vi "RT_VS50_Dynamics_DLR_v10_v11_PXI.vi"() -> ()   [LabVIEW 2017]
uses:
  <vilib>/Platform/TimedLoop/XDataNode/timing_clust.ctl
  <vilib>/Platform/TimedLoop/XDataNode/nitl_modes.ctl
  <vilib>/Platform/TimedLoop/XDataNode/wakeup.ctl
  <vilib>/Analysis/coordinate.llb/Euler Rotation Order.ctl
  <vilib>/Analysis/_algsub.llb/Vector Norm Type.ctl
  <vilib>/Analysis/baseanly.llb/Real A x B.vi
  <vilib>/Analysis/_algsub.llb/Real Vector Norm.vi
  <vilib>/Utility/file.llb/Read Delimited Spreadsheet (DBL).vi
  <vilib>/Instr/_visa.llb/VISA Configure Serial Port (Instr).vi
  <vilib>/Analysis/Matrix/Numeric/Conversions/Array To Matrix - RA.vi
  <vilib>/Analysis/Matrix/Numeric/Conversions/Array To Matrix - RA2.vi
  <vilib>/Analysis/Matrix/Numeric/Conversions/Matrix To Array - RM.vi
  <vilib>/Platform/TimedLoop/XDataNode/XDataNode.xnode
  <vilib>/Analysis/NI_AALPro.lvlib
  <vilib>/Platform/TimedLoop/XDataNode/XDNodeRunTimeDep.lvlib
  <vilib>/Utility/file.llb/Read From Spreadsheet File (DBL).vi
  <vilib>/Analysis/Matrix/NI_Matrix.lvlib
  <vilib>/Analysis/NI_AALBase.lvlib
panel:
  out "Sim_Time [s]":dbl
  in  "Simulation Parameters":T1={"Wind VelocityAzimuth [deg] "=0.0, "Wind Velocity Module [m/s]"=0.0, "Fe gain"=1.0, "Cnalpha gain"=1.0, "clp gain"=1.0, "cld gain"=1.0, "cmq gain"=1.0, "cnr gain"=1.0, "dl [º]"=0.0, "Nozzle misalignment yaw/pitch [º]"=[0.0, 0.0], "Nozzle eccentricity x/y [m]"=[], "Wind_Profile"=0} {"Wind_Profile" min=0 max=3 step=1; "Wind Velocity Module [m/s]" format="%#_13g"; "Wind VelocityAzimuth [deg]" format="%#_13g"}
  in  "Initialization Parameters":T2={"W_b ini [rad/s]"=[0.0, 0.0, 0.0], "W ini [rad/s]"=[0.0, 0.0, 0.0], "altitude_ini(m)"=50.0, "lon_ini [º]"=-44.36778, "latd_ini [º]"=-2.31599, "V_ini [m/s]"=[0.0, 0.0, 0.0], "Initial Euler Angles [deg]"=[0.0, 0.0, 0.0], "CFN-61G Enable"=FALSE, "Table enable"=FALSE, "DMARS Enable"=FALSE, "TVA Enable"=FALSE, "Sim_Time [s]"=82.0, "Control Selection"=enum."Sim Control"}
  in  "Rotation":T3
  out "Initial Euler Angles [deg] 2":cluster{"phi":dbl, "theta":dbl, "psi":dbl}
  out "TVA_cmd [deg] 2":dbl[](array[numeric])
  out "Control Variables (extra variables)":dbl[](array[numeric])
  in  "Send":bool
  out "Table Ready":bool
  out "CIVITA as DMARS [º]":cluster{"phi":dbl, "theta":dbl, "psi":dbl}
  in  "Cluster":T4={"Offset Roll"=0.0, "Offset Pitch"=0.0, "Offset Heading"=0.0, "Azimuth"=0.0, "Latitude "=-23.213156, "Longitude"=-45.860622, "Height"=622.367, "LP_Vel_Z-North"=0.0, "LP_Vel_Y-East"=0.0, "LP_Vel_X-Up"=0.0}
  out "Table cmd [º] inner middle outer":dbl[](array[numeric])
  out "DMARS SIM pred[º]":cluster{"phi":dbl, "theta":dbl, "psi":dbl}
  out "Control Variables\n (extra variables)":dbl[](array[numeric])
  out "ACT 315 Angle \"Yaw\"":dbl(slide) scale=-3.0..3.0
  out "ACT 225 Angle \"Pitch\"":dbl(slide) scale=-3.0..3.0
  out "TVA string 2":string
  out "TVA bytes read 2":u32
  out "CRC Check over Byte #10 to byte #84":bool
  out "CRC Check over Byte #2 to Byte #7 TVA2BComp":bool
  out "Iteration Duration":i64
  out "Roll Rate/angle":dbl[](array[numeric])
  out "CRC Check over Byte #2 to Byte #7":bool
  out "CRC Check over Byte #10 to byte #29":bool
  out "GC_Counter 2":u32
  out "concatenated string 2":string
  out "PXI log path 2":path
  out "string to write DMARS":string="*IDN?"
  out "TVA string":string
  out "TVA bytes read":u32
  out "TVA sync bytes":string
  out "read buffer":string
  out "concatenated string":string
  out "appended path":path
  in  "UTC format":bool
  out "spreadsheet string":string
  out "Time (s)":dbl
  out "POS":cluster{dbl, dbl, dbl} {"?" format="%_6g"; "?" format="%#1_6g"}
  out "RATE":cluster{dbl, dbl, dbl} {"?" format="%1_6g"}
  out "ACCEL":cluster{dbl, dbl, dbl} {"?" format="%1_6g"}
  out "Period":i64
  in  "predicted step":dbl=0.04 format="%#_13g"
  out "string enviada para acutrol":string
  in  "Remote Host":string="192.168.53.1"
  out "XYZ - rate_CIVITA":sgl[](array[numeric])
  out "Opp_Mode_CIVITA":string
  in  "NavOn":bool
  in  "Init":bool
  out "read Config port":string
  out "Long_Lat_Alt_CIVITA":sgl[](array[numeric])
  out "Euler Angles_CIVITA":sgl[](array[numeric])
  out "all rows":dbl[][](array[numeric]) format="%0.3f"
  in  "Run_SIMULATION":bool
  out "Data 4":dbl[][](array[numeric])
  out "Data 3":dbl[][](array[numeric])
  out "Data 2":dbl[][](array[numeric])
  out "Iteration Duration [us]":i64(graph)
  out "Current time [s]":dbl
  out "TVA_cmd [deg]":dbl[](array[numeric])
  out "bad iteration":bool
  in  "stop RT":bool
  out "SIM_Running":bool
  # "atitudes após leveling"
  # "INS Civitanavi Control"
  # "0.279817"
  # "0.24729"
  # "0.119821"
  # "-0.038247"
  # "0xAA/ 0x55"
  # "-0.038932"
  # "-0.0385253"
  # "-0.0178696"
  # "-0.0193609"
  # "-0.0176574"
  # "830 steps"
  # "Posicão inicial"
  # "Posicao after 10min"
  # "-48.1427"
  # "-45.8606"
  # "-23.2324"
  # "-23.2132"
  # "-4.67869"
  # "0.622374"
  # "º"
  # "º"
  # "Km"
  # "Simulation"
  # "Motion simulation table Control and Log files"
  # "Reiniciar a vi sempre antes de uma nova simulação!!"
  # "0.766"
  # "1.532"
  # "Enable buttons"
  # "TVA COMMUNICATIONS"
  # "0.643"
  # "1.286"
  # "Housekeeping data"
  # "Command Data"
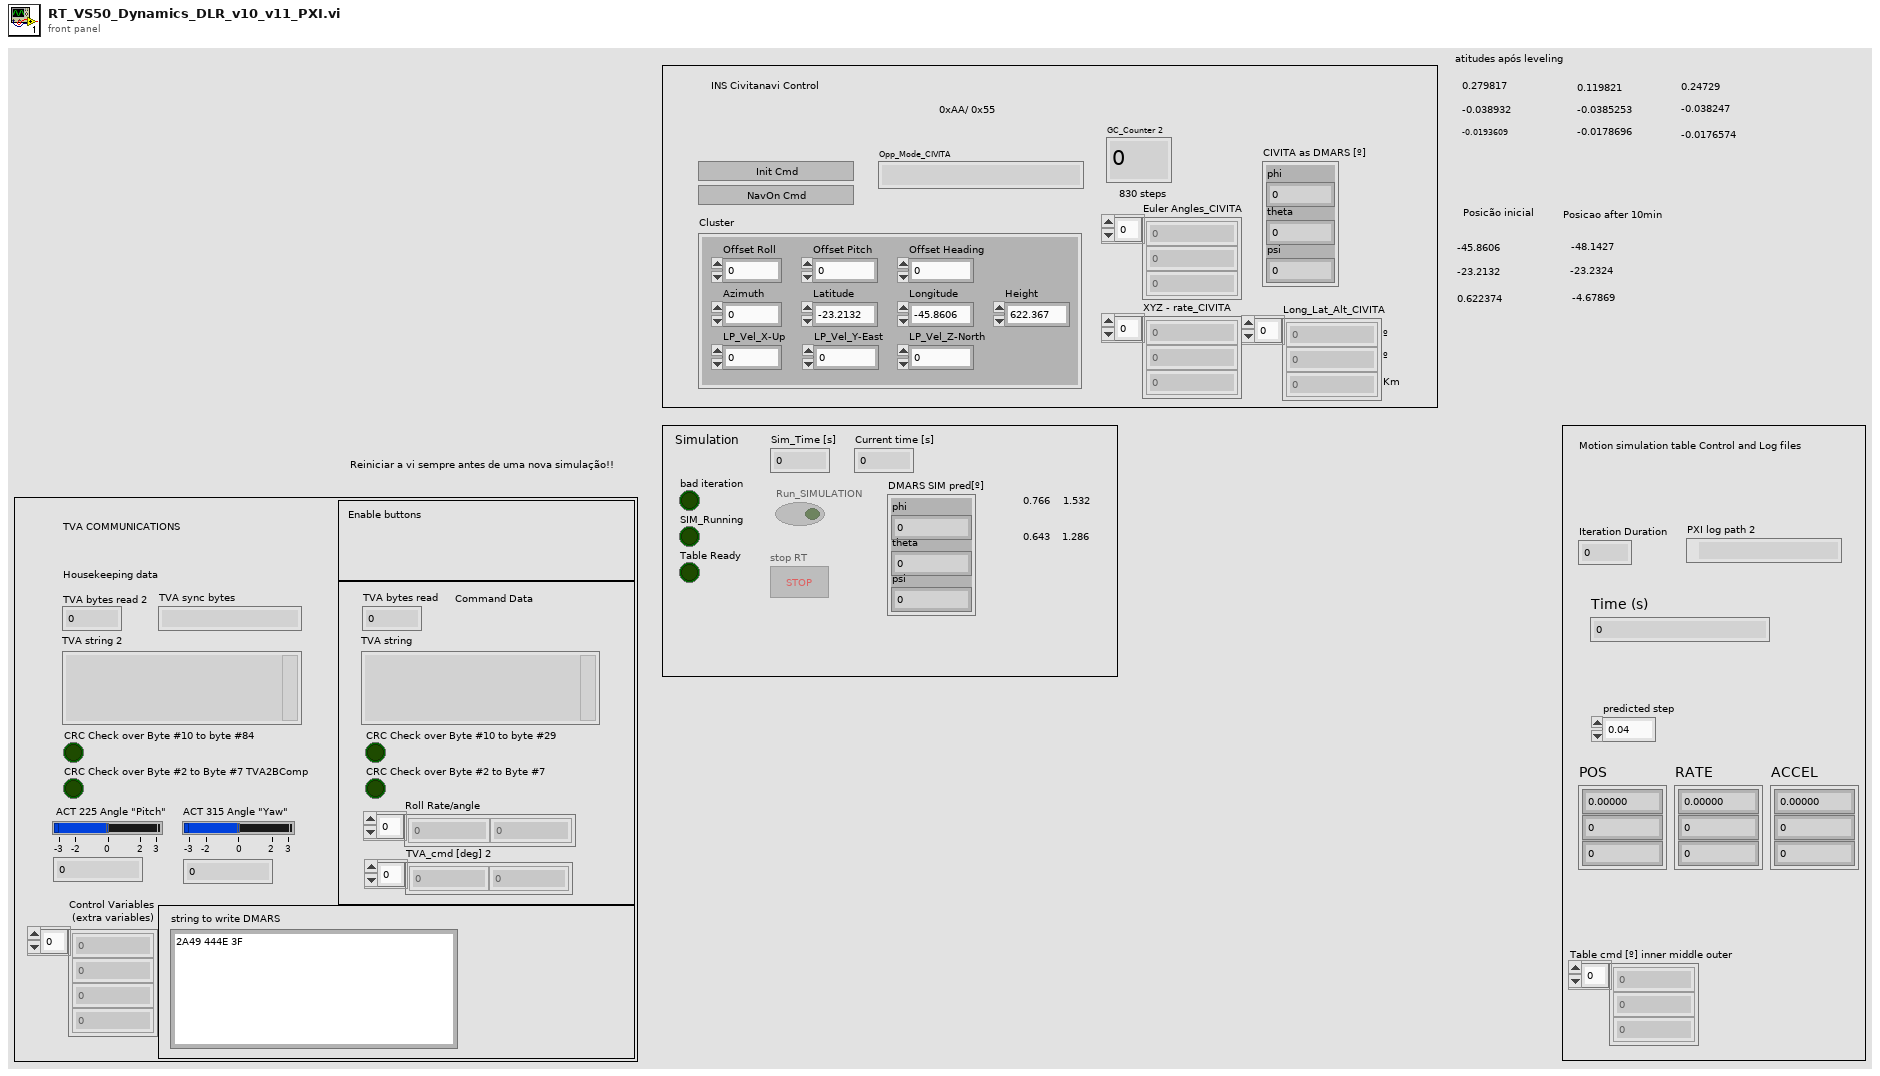
[diagram p1: front panel]
types:
  T1 = cluster{"Wind VelocityAzimuth [deg] ":dbl, "Wind Velocity Module [m/s]":dbl, "Fe gain":dbl, "Cnalpha gain":dbl, "clp gain":dbl, "cld gain":dbl, "cmq gain":dbl, "cnr gain":dbl, "dl [º]":dbl, "Nozzle misalignment yaw/pitch [º]":dbl[], "Nozzle eccentricity x/y [m]":dbl[], "Wind_Profile":i32}
  T2 = cluster{"W_b ini [rad/s]":dbl[], "W ini [rad/s]":dbl[], "altitude_ini(m)":dbl, "lon_ini [º]":dbl, "latd_ini [º]":dbl, "V_ini [m/s]":dbl[], "Initial Euler Angles [deg]":dbl[], "CFN-61G Enable":bool, "Table enable":bool, "DMARS Enable":bool, "TVA Enable":bool, "Sim_Time [s]":dbl, "Control Selection":enum16{"Constant", "TVA E-BOX", "Sim Control"}}
  T3 = cluster{"W(i) [rad/s]":dbl[], "W_b(i) [rad/s]":dbl[], "q(i)":dbl[], "Euler Angles {rad]":dbl[]}
  T4 = cluster{"Offset Roll":sgl, "Offset Pitch":sgl, "Offset Heading":sgl, "Azimuth":sgl, "Latitude ":sgl, "Longitude":sgl, "Height":sgl, "LP_Vel_Z-North":sgl, "LP_Vel_Y-East":sgl, "LP_Vel_X-Up":sgl}
  T5 = typedef "XDNodeRunTimeDep.lvlib/timing_clust.ctl" = cluster{"Expected End [f-1]":u64, "Actual End [f-1]":u64, "Finished Late? [f-1]":bool, "Expected End [i-1]":u64, "Actual End [i-1]":u64, "Finished Late? [i-1]":bool, "Expected Start [i]":u64, "Actual Start [i]":u64, "Expected Start [f]":u64, "Actual Start [f]":u64, "Source Name":string, "Structure Name":string, "Period":i64, "Deadline":i64, "Offset":i64, "Start":i64, "Priority":i32, "Timeout":i32, "Mode":T6, "Wakeup Reason":T7, "Error":errorcluster, "Source Type":string, "Secondary Source Type":string, "Global End Time":u64, "Global Start Time":u64, "Frame Duration":u64, "Iteration Duration":u64, "Assigned CPU":i32, "I/O Scan Engine Mode":u32}
  T6 = typedef "XDNodeRunTimeDep.lvlib/nitl_modes.ctl" = enum32{"No Change", "Process missed periods, maintain original phase", "Discard missed periods, maintain original phase", "Process missed periods, ignore original phase", "Discard missed periods, ignore original phase"}
  T7 = typedef "XDNodeRunTimeDep.lvlib/wakeup.ctl" = enum32{"Normal", "Aborted", "Asynchronous wakeup", "Timing source error", "Timed loop error", "Timeout"}
  T8 = cluster{"act_b [rad]":dbl[], "Oil Consumption [L]":dbl, "Act_b_TVA (315,225) [deg]":dbl[]}
  T9 = cluster{"W(i+1) [rad/s]":dbl[], "W_b(i+1) [rad/s]":dbl[], "q(i+1)":dbl[], "Euler angles (i+1) XYZ [rad]":dbl[]}
  T10 = cluster{"position ECEF (i)":dbl[], "Lat_C [rad]":dbl, "latd(i+1) [rad]":dbl, "lon(i+1) [rad]":dbl, "height (i+1) [m]":dbl, "V(i+1) [m/s] NWU":dbl[]}
  T11 = cluster{"latd(i) [rad]":dbl, "lon(i) [rad]":dbl, "height(i)(m)":dbl, "V(i) [m/s] NWU":dbl[]}
  T12 = typedef "NI_AALPro.lvlib/Euler Rotation Order.ctl" = u16
  T13 = cluster{"dt [s]":dbl, "sim_running":bool, "t[s]":dbl, "i":i32}
  T14 = cluster{"Nzl_S [m^2]":dbl, "le [m]":dbl, "dl [rad]":dbl, "Dref[m]":dbl, "Sref [m^2]":dbl, "Nozzle misalignment yaw/pitch [º]":dbl[], "Nozzle eccentricity x/y [m]":dbl[]}
  T15 = typedef "NI_Matrix.lvlib/RealMatrix.ctl" = dbl[][]
  T16 = cluster{"AoA_pitch [rad]":dbl, "AoA_yaw [rad]":dbl, "Stream_direction [rad]":dbl[], "Speed_direction [rad]":dbl[]}
  T17 = cluster{"M_alpha [rad/s²]":dbl, "M_beta [rad/s²]":dbl}
  T18 = typedef "NI_AALPro.lvlib/Vector Norm Type.ctl" = u16
  T19 = enum16{"open", "replace", "create", "open or create", "replace or create", "replace or create with confirmation"}
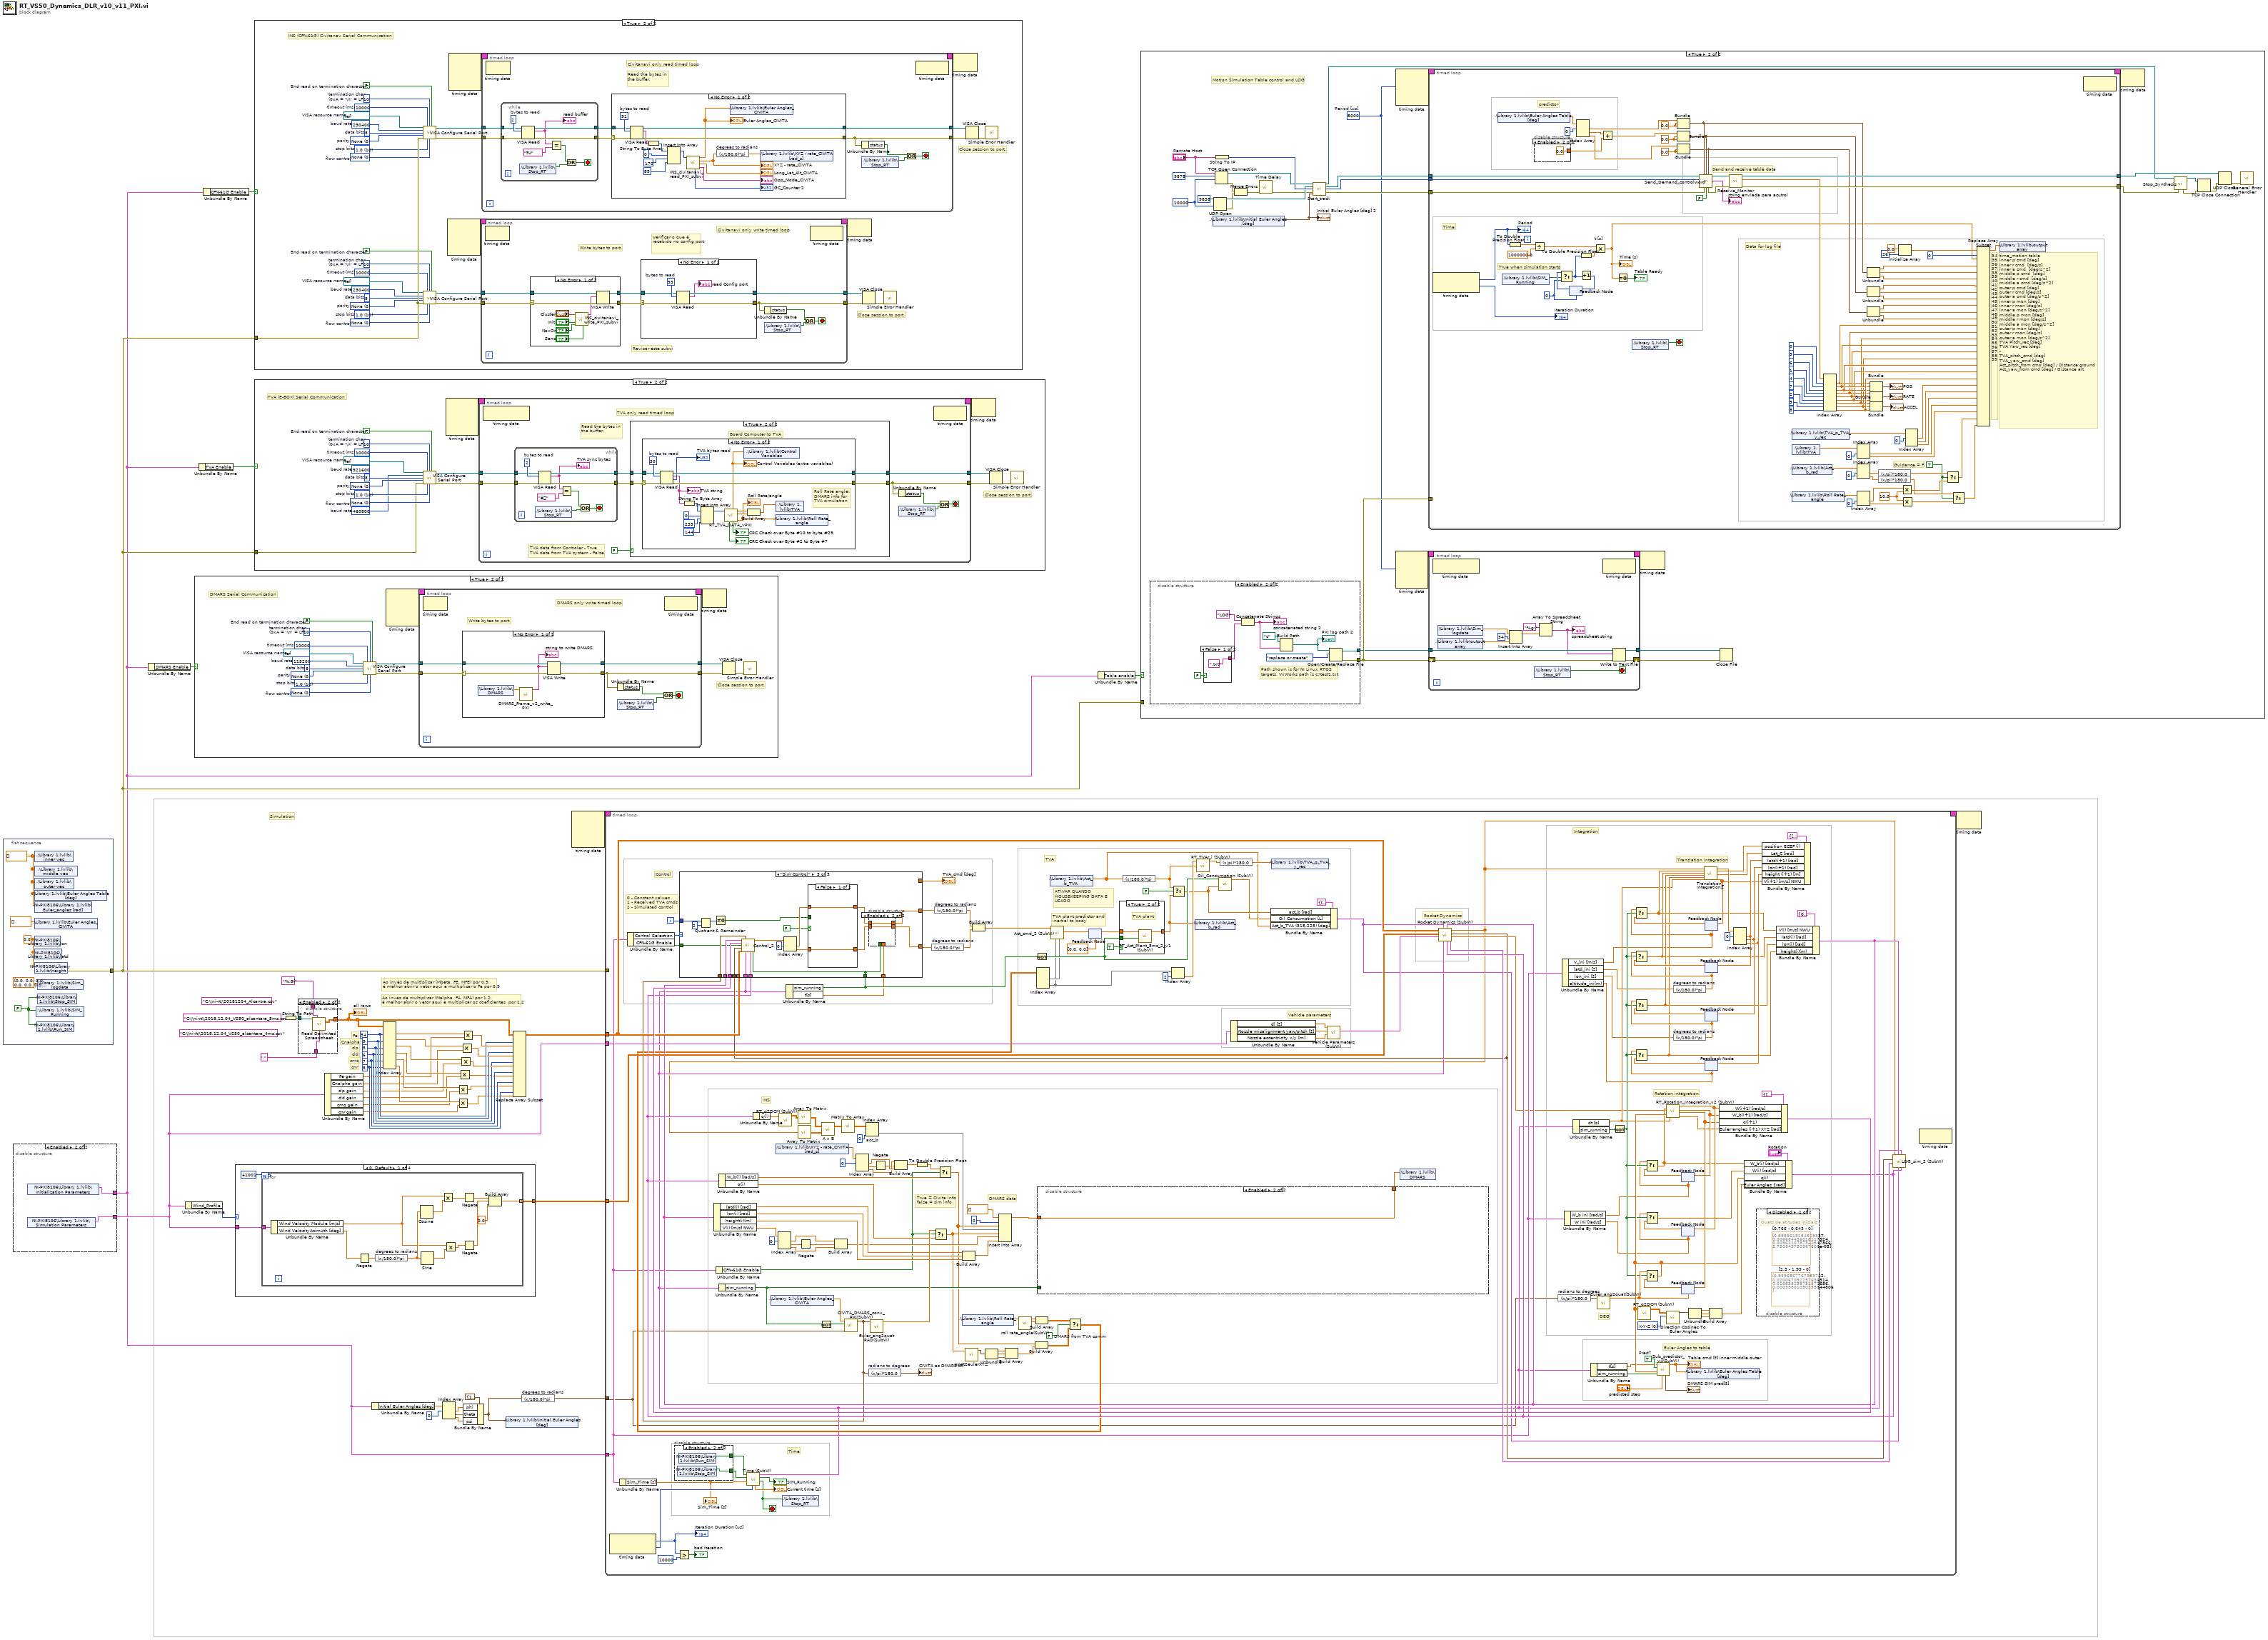
[diagram p0: block diagram]
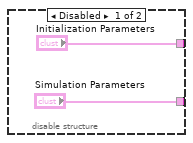
[diagram p2: hidden frame]
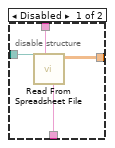
[diagram p3: hidden frame]
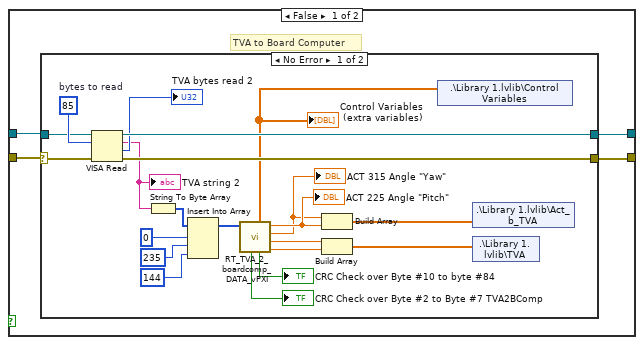
[diagram p11: hidden frame]
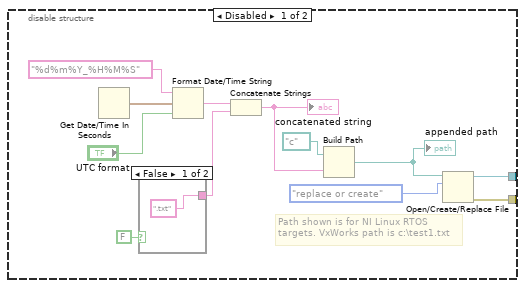
[diagram p15: hidden frame]
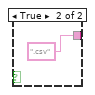
[diagram p16: hidden frame]
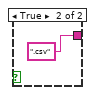
[diagram p17: hidden frame]
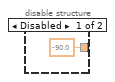
[diagram p18: hidden frame]
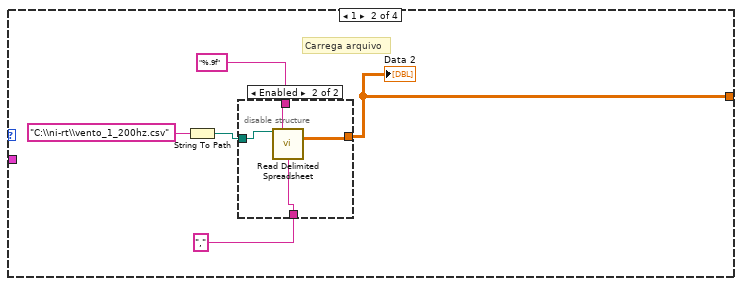
[diagram p19: hidden frame]
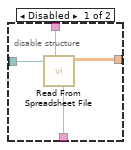
[diagram p20: hidden frame]
diagram:
  w27 = 8 ("index (col)")
  w28 = 7 ("index (col)")
  w29 = 6 ("index (col)")
  w33 = 5 ("index (col)")
  w36 = 9 ("index (col)")
  w41 = 54 ("disabled index (col)")
  (unwired) "C:\\ni-rt\\2018.12.04_VS50_alcantara_4ms.csv"
  (unwired) "C:\\ni-rt\\20181204_Alcantra.csv"
  # "cnr"
  # "cmq"
  # "cld"
  # "clp"
  # "Cnalpha"
  # "Fe"
  # "Ao invés de multiplicar (Malpha, FA, MFA) por 1.2,\né melhor abrir o vetor aqui e multiplicar os coeficientes  por 1.2"
  # "Ao invés de multiplicar (Mbeta, FE, MFE) por 0.9,\né melhor abrir o vetor aqui e multiplicar o Fe por 0.9"
  # "Simulation"
  n1 = flat-sequence {
    tunnel: [w53] -> w22
    frame #0 {
      w52 = dbl[] [] ("inner vec")
      w50 = FALSE ("SIM_Running")
      w55 = 0.0 ("lon")
      n2 = shared-variable ".\\Library 1.lvlib\\inner vec"(w52) -> ()  [unwired: 1 in, 1 out]
      n3 = shared-variable ".\\Library 1.lvlib\\middle vec"(w52) -> ()  [unwired: 1 in, 1 out]
      n4 = shared-variable ".\\Library 1.lvlib\\outer vec"(w52) -> ()  [unwired: 1 in, 1 out]
      n5 = shared-variable ".\\Library 1.lvlib\\Euler Angles Table [deg]"(w52) -> ()  [unwired: 1 in, 1 out]
      n6 = shared-variable "NI-PXI8106\\Library 1.lvlib\\Euler_angles [rad]"(w52) -> ()  [unwired: 1 in, 1 out]
      n7 = shared-variable ".\\Library 1.lvlib\\Euler Angles_CIVITA"(sgl[] [] ("Euler Angles_CIVITA")) -> ()  [unwired: 1 in, 1 out]
      n8 = shared-variable "NI-PXI8106\\Library 1.lvlib\\lon"(w55) -> ()  [unwired: 1 in, 1 out]
      n9 = shared-variable "NI-PXI8106\\Library 1.lvlib\\latd"(w55) -> ()  [unwired: 1 in, 1 out]
      n10 = shared-variable "NI-PXI8106\\Library 1.lvlib\\height"(w55) -> (error out=w53:errorcluster)  [unwired: 1 in]
      n11 = shared-variable ".\\Library 1.lvlib\\SIM_Running"(w50) -> ()  [unwired: 1 in, 1 out]
      n12 = shared-variable "NI-PXI8106\\Library 1.lvlib\\Run_SIM"(w50) -> ()  [unwired: 1 in, 1 out]
      n13 = shared-variable ".\\Library 1.lvlib\\Sim_logdata"(dbl[] [0.0, 0.0, 0.0, 0.0, 0.0, 0.0, 0.0, 0.0, 0.0, 0.0, 0.0, 0.0, 0.0, 0.0, 0.0, 0.0, 0.0, 0.0, 0.0, 0.0, 0.0, 0.0, 0.0, 0.0, 0.0, 0.0, 0.0, 0.0, 0.0, 0.0, 0.0, 0.0, 0.0] ("Sim_logdata")) -> ()  [unwired: 1 in, 1 out]
      n14 = shared-variable "NI-PXI8106\\Library 1.lvlib\\Stop_SIM"(w50) -> ()  [unwired: 1 in, 1 out]
    }
  }
  n15 = disable-structure shown="Enabled" {
    disable-tunnel: ["Initialization Parameters" w58] -> w1
    disable-tunnel: ["Simulation Parameters" w59] -> w4
    frame Disabled {
    }
    frame Enabled {
      n16 = shared-variable "NI-PXI8106\\Library 1.lvlib\\Simulation Parameters"() -> (w59:T1)  [unwired: 1 in, 1 out]
      n17 = shared-variable "NI-PXI8106\\Library 1.lvlib\\Initialization Parameters"() -> (w58:T2)  [unwired: 1 in, 1 out]
    }
  }
  n18 = Unbundle By Name(w1) -> ("DMARS Enable"=w15:bool)
  n19 = Unbundle By Name(w4) -> ("Wind_Profile"=w11:i32)
  n20 = case shown="True" w15 {
    frame False {
    }
    frame True {
      w68 = u32 10000  # timeout (ms)
      w65 = u16 0 items=["None"=0, "XON/XOFF"=1, "RTS/CTS"=2, "DTR/DSR"=4]  # flow control
      w69 = u16 10 items=["1.0"=10, "1.5"=15, "2.0"=20]  # stop bits
      w70 = u16 0 items=["None", "Odd", "Even", "Mark", "Space"]  # parity
      w67 = FALSE  # End read on termination character?
      w66 = u8 10  # termination char (0xA = '\n' = LF)
      w64 = u16 8  # data bits
      w73 = u32 115200  # baud rate
      w72 = refnum<visa-resource-name> "COM3"  # VISA resource name
      # "DMARS Serial Communication"
      # "Close session to port."
      n21 = call-poly "VISA Configure Serial Port"("VISA resource name"=w72, "timeout (10sec)"=w68, "termination char\n(0xA = '\\n' = LF)"=w66, "Enable Termination\nChar (T)"=w67, "baud rate (9600)"=w73, "data bits (8)"=w64, "parity (0:none)"=w70, "stop bits (10: 1 bit)"=w69, "flow control (0:none)"=w65) -> ("VISA resource name out"=w61:refnum<visa-resource-name>, "error out"=w60:errorcluster)  [unwired: 1 in, 4 out]
      n22 = node-c288() -> (w75:T5)  [unwired: 4 in]
      n23 = timed-loop {
        tunnel: w60 -> [w80]
        tunnel: w61 -> [w81]
        tunnel: [w77] -> w63
        tunnel: [w76] -> w62
        timing: w75 -> [_]
        timing-out: [_] -> w74
        stop <- w79 stop-if-true
        # "Write bytes to port."
        # "DMARS only write timed loop"
        n24 = node-c288() -> ()  [unwired: 1 in, 1 out]
        n25 = case shown="No Error" w80 {
          selector: w80 -> [w85 w90]
          tunnel: [w88 w89] -> w77
          tunnel: [w87 w90] -> w76
          tunnel: w81 -> [w86 w89]
          frame No Error {
            n26 = shared-variable ".\\Library 1.lvlib\\DMARS"() -> (w84:dbl[])  [unwired: 1 in, 1 out]
            n27 = call "DMARS_Frame_v2_write_PXI.vi"("DMARS"=w84) -> ("string_Out"=w83:string)  [unwired: 9 in, 1 out]
            "string to write DMARS" <- w83
            n28 = VISA Write(VISA resource name=w86, write buffer=w83, error in (no error)=w85) -> (VISA resource name out=w88:refnum<visa-resource-name>, error out=w87:errorcluster)  [unwired: 1 out]
          }
          frame Error {
          }
        }
        n29 = Unbundle By Name(w76) -> ("status"=w82:bool)
        n30 = shared-variable ".\\Library 1.lvlib\\Stop_RT"() -> (w78:bool)  [unwired: 1 in, 1 out]
        n31 = Or(x=w82, y=w78) -> (x .or. y?=w79:bool)
        n32 = node-c288() -> ()  [unwired: 1 in, 1 out]
      }
      n33 = node-c288(w74) -> ()  [unwired: 1 out]
      n34 = VISA Close(VISA resource name=w63, error in (no error)=w62) -> (error out=w71:errorcluster)
      n35 = call <vilib>:"Simple Error Handler.vi"("error in (no error)"=w71) -> ()  [unwired: 1 in, 8 out]
    }
  }
  n36 = Unbundle By Name(w1) -> ("TVA Enable"=w14:bool)
  n37 = Unbundle By Name(w1) -> ("CFN-61G Enable"=w13:bool)
  n38 = case shown="0, Default" w11 {
    tunnel: [w96 w111 w124 w137] -> w45
    tunnel: w4 -> [w95 _ _ _]
    frame 0, Default {
      n39 = for {
        N: 41001 -> [_]
        tunnel: [w110] -> w96 mode=indexing
        tunnel: w95 -> [w100]
        n40 = Unbundle By Name(w100) -> ("Wind Velocity Module [m/s]"=w99:dbl, "Wind VelocityAzimuth [deg]"=w98:dbl)
        n41 = Negate(x=w98) -> (-x=w101:dbl)
        n42 = expression code="(x/180.0)*pi" "degrees to radians"(w101) -> (w102:dbl)
        n43 = Cosine(x=w102) -> (cos(x)=w108:dbl)
        n44 = Sine(x=w102) -> (sin(x)=w105:dbl)
        n45 = Multiply(x=w99, y=w108) -> (x*y=w107:dbl)
        n46 = Multiply(x=w99, y=w105) -> (x*y=w104:dbl)
        n47 = Negate(x=w107) -> (-x=w106:dbl)
        n48 = Negate(x=w104) -> (-x=w103:dbl)
        n49 = Build Array(w106, w103, 0.0 ("element")) -> (w110:dbl[])
      }
    }
    frame 1 {
      # "Carrega arquivo"
      n50 = String To Path(string="C:\\ni-rt\\vento_1_200hz.csv") -> (path=w114:path)
      n51 = disable-structure shown="Enabled" {
        disable-tunnel: "%.9f" ("format (%.3f)") -> [w119 w123]
        disable-tunnel: w114 -> [w118 w122]
        disable-tunnel: "," ("delimiter (\\t)") -> [w117 w120]
        disable-tunnel: [w116 w121] -> w111
        frame Disabled {
          n52 = call-poly <vilib>:"Read From Spreadsheet File.vi"("delimiter (\\t)"=w117, "format (%.3f)"=w119, "file path (dialog if empty)"=w118) -> ("all rows"=w116:dbl[][])  [unwired: 4 in, 4 out]
        }
        frame Enabled {
          n53 = call-poly <vilib>:"Read Delimited Spreadsheet.vi"("file path (dialog if empty)"=w122, "format (%.3f)"=w123, "delimiter (\\t)"=w120) -> ("all rows"=w121:dbl[][])  [unwired: 7 in, 5 out]
        }
      }
      "Data 2" <- w111
    }
    frame 2 {
      # "Carrega arquivo"
      n54 = String To Path(string="C:\\ni-rt\\vento_2_200hz.csv") -> (path=w127:path)
      n55 = disable-structure shown="Enabled" {
        disable-tunnel: "%.9f" ("format (%.3f)") -> [w132 w136]
        disable-tunnel: w127 -> [w131 w135]
        disable-tunnel: "," ("delimiter (\\t)") -> [w130 w133]
        disable-tunnel: [w129 w134] -> w124
        frame Disabled {
          n56 = call-poly <vilib>:"Read From Spreadsheet File.vi"("delimiter (\\t)"=w130, "format (%.3f)"=w132, "file path (dialog if empty)"=w131) -> ("all rows"=w129:dbl[][])  [unwired: 4 in, 4 out]
        }
        frame Enabled {
          n57 = call-poly <vilib>:"Read Delimited Spreadsheet.vi"("file path (dialog if empty)"=w135, "format (%.3f)"=w136, "delimiter (\\t)"=w133) -> ("all rows"=w134:dbl[][])  [unwired: 7 in, 5 out]
        }
      }
      "Data 3" <- w124
    }
    frame 3 {
      # "Carrega arquivo"
      n58 = String To Path(string="C:\\ni-rt\\vento_4_200hz.csv") -> (path=w139:path)
      n59 = disable-structure shown="Enabled" {
        disable-tunnel: "%.9f" ("format (%.3f)") -> [w145 w149]
        disable-tunnel: w139 -> [w144 w148]
        disable-tunnel: "," ("delimiter (\\t)") -> [w143 w146]
        disable-tunnel: [w142 w147] -> w137
        frame Disabled {
          n60 = call-poly <vilib>:"Read From Spreadsheet File.vi"("delimiter (\\t)"=w143, "format (%.3f)"=w145, "file path (dialog if empty)"=w144) -> ("all rows"=w142:dbl[][])  [unwired: 4 in, 4 out]
        }
        frame Enabled {
          n61 = call-poly <vilib>:"Read Delimited Spreadsheet.vi"("file path (dialog if empty)"=w148, "format (%.3f)"=w149, "delimiter (\\t)"=w146) -> ("all rows"=w147:dbl[][])  [unwired: 7 in, 5 out]
        }
      }
      "Data 4" <- w137
    }
  }
  n62 = case shown="True" w13 {
    tunnel: w22 -> [_ w178]
    frame False {
    }
    frame True {
      w156 = u32 10000  # timeout (ms)
      w158 = u16 0 items=["None"=0, "XON/XOFF"=1, "RTS/CTS"=2, "DTR/DSR"=4]  # flow control
      w155 = u16 10 items=["1.0"=10, "1.5"=15, "2.0"=20]  # stop bits
      w154 = u16 0 items=["None", "Odd", "Even", "Mark", "Space"]  # parity
      w150 = FALSE  # End read on termination character?
      w157 = u8 10  # termination char (0xA = '\n' = LF)
      w159 = u16 8  # data bits
      w151 = u32 230400  # baud rate
      w152 = refnum<visa-resource-name> "COM4"  # VISA resource name
      w172 = u32 10000  # timeout (ms)
      w169 = u16 0 items=["None"=0, "XON/XOFF"=1, "RTS/CTS"=2, "DTR/DSR"=4]  # flow control
      w173 = u16 10 items=["1.0"=10, "1.5"=15, "2.0"=20]  # stop bits
      w174 = u16 0 items=["None", "Odd", "Even", "Mark", "Space"]  # parity
      w171 = FALSE  # End read on termination character?
      w170 = u8 10  # termination char (0xA = '\n' = LF)
      w168 = u16 8  # data bits
      w177 = u32 230400  # baud rate
      w176 = refnum<visa-resource-name> "COM3"  # VISA resource name
      # "INS (CFN-61G) Civitanav Serial Communication"
      # "Close session to port."
      # "Close session to port."
      n63 = call-poly "VISA Configure Serial Port"("VISA resource name"=w176, "timeout (10sec)"=w172, "termination char\n(0xA = '\\n' = LF)"=w170, "Enable Termination\nChar (T)"=w171, "baud rate (9600)"=w177, "data bits (8)"=w168, "parity (0:none)"=w174, "error in (no error)"=w178, "stop bits (10: 1 bit)"=w173, "flow control (0:none)"=w169) -> ("VISA resource name out"=w165:refnum<visa-resource-name>, "error out"=w164:errorcluster)  [unwired: 4 out]
      n64 = call-poly "VISA Configure Serial Port"("VISA resource name"=w152, "timeout (10sec)"=w156, "termination char\n(0xA = '\\n' = LF)"=w157, "Enable Termination\nChar (T)"=w150, "baud rate (9600)"=w151, "data bits (8)"=w159, "parity (0:none)"=w154, "error in (no error)"=w178, "stop bits (10: 1 bit)"=w155, "flow control (0:none)"=w158) -> ("VISA resource name out"=w162:refnum<visa-resource-name>, "error out"=w163:errorcluster)  [unwired: 4 out]
      n65 = node-c288() -> (w180:T5)  [unwired: 4 in]
      n66 = node-c288() -> (w182:T5)  [unwired: 4 in]
      n67 = timed-loop {
        tunnel: w163 -> [w187]
        tunnel: w162 -> [w188]
        tunnel: [w186] -> w160
        tunnel: [w185] -> w161
        timing: w180 -> [_]
        timing-out: [_] -> w179
        stop <- w184 stop-if-true
        # "Revisar este subvi"
        # "Verificar o que é recebido no config port"
        # "Write bytes to port."
        # "Civitanavi only write timed loop"
        n68 = node-c288() -> ()  [unwired: 1 in, 1 out]
        n69 = case shown="No Error" w187 {
          selector: w187 -> [w205 w210]
          tunnel: [w208 w209] -> w190
          tunnel: [w207 w210] -> w189
          tunnel: w188 -> [w206 w209]
          frame No Error {
            n70 = call "INS_civitanavi_write_PXI_subvi.vi"("Send"="Send", "NavOn"="NavOn", "Init"="Init", "Cluster"="Cluster") -> ("string out"=w204:string)  [unwired: 7 in]
            n71 = VISA Write(VISA resource name=w206, write buffer=w204, error in (no error)=w205) -> (VISA resource name out=w208:refnum<visa-resource-name>, error out=w207:errorcluster)  [unwired: 1 out]
          }
          frame Error {
          }
        }
        n72 = case "Read bytes from port." shown="No Error" w189 {
          selector: w189 -> [w193 w198]
          tunnel: [w196 w198] -> w185
          tunnel: [w197 w199] -> w186
          tunnel: w190 -> [w194 w199]
          frame No Error {
            w195 = u32 93  # bytes to read
            n73 = VISA Read(VISA resource name=w194, byte count=w195, error in (no error)=w193) -> (VISA resource name out=w197:refnum<visa-resource-name>, read buffer=→"read Config port":string, error out=w196:errorcluster)  [unwired: 1 out]
          }
          frame Error {
            # "Error occurred \nreading Bytes at \nSerial Port"
          }
        }
        n74 = Unbundle By Name(w185) -> ("status"=w191:bool)
        n75 = shared-variable ".\\Library 1.lvlib\\Stop_RT"() -> (w183:bool)  [unwired: 1 in, 1 out]
        n76 = Or(x=w191, y=w183) -> (x .or. y?=w184:bool)
        n77 = node-c288() -> ()  [unwired: 1 in, 1 out]
      }
      n78 = timed-loop {
        tunnel: w164 -> [w219]
        tunnel: w165 -> [w220]
        tunnel: [w218] -> w167
        tunnel: [w217] -> w166
        timing: w182 -> [_]
        timing-out: [_] -> w181
        stop <- w216 stop-if-true
        # "Read the bytes in the buffer."
        # "Civitanavi only read timed loop"
        n79 = node-c288() -> ()  [unwired: 1 in, 1 out]
        n80 = while {
          tunnel: w220 -> [w251]
          tunnel: w219 -> [w250]
          tunnel: [w249] -> w222
          tunnel: [w248] -> w221
          stop <- w243 stop-if-true
          w252 = u32 2  # bytes to read
          n81 = shared-variable ".\\Library 1.lvlib\\Stop_RT"() -> (w245:bool)  [unwired: 1 in, 1 out]
          n82 = VISA Read(VISA resource name=w251, byte count=w252, error in (no error)=w250) -> (VISA resource name out=w249:refnum<visa-resource-name>, read buffer=w247:string, error out=w248:errorcluster)  [unwired: 1 out]
          "read buffer" <- w247
          n83 = Equal?(x=w247, y="ªU") -> (x = y?=w244:bool)
          n84 = Or(x=w244, y=w245) -> (x .or. y?=w243:bool)
        }
        n85 = case "Read bytes from port." shown="No Error" w221 {
          selector: w221 -> [w236 w241]
          tunnel: [w239 w241] -> w217
          tunnel: [w240 w242] -> w218
          tunnel: w222 -> [w237 w242]
          frame No Error {
            w238 = u32 91  # bytes to read
            n86 = VISA Read(VISA resource name=w237, byte count=w238, error in (no error)=w236) -> (VISA resource name out=w240:refnum<visa-resource-name>, read buffer=w235:string, error out=w239:errorcluster)  [unwired: 1 out]
            n87 = String To Byte Array(string=w235) -> (unsigned byte array=w231:u8[])
            n88 = Insert Into Array(array=w231, index=0, new element #1=u8 170 ("new element/subarray"), new element #2=u8 85 ("new element/subarray")) -> (w230:u8[])
            n89 = call "INS_civitanavi_read_PXI_subvi.vi"("U8_Input"=w230) -> ("Opp_Mode 2"=→"Opp_Mode_CIVITA":string, "Long_Lat_Alt"=→"Long_Lat_Alt_CIVITA":sgl[], "XYZ - rate"=w224:sgl[], "Euler Angles"=w234:sgl[], "GC_Counter 2"=→"GC_Counter 2":u32)  [unwired: 6 in]
            "Euler Angles_CIVITA" <- w234
            "XYZ - rate_CIVITA" <- w224
            n90 = expression code="(x/180.0)*pi" "degrees to radians"(w224) -> (w225:sgl[])
            n91 = shared-variable ".\\Library 1.lvlib\\Euler Angles_CIVITA"(w234) -> ()  [unwired: 1 in, 1 out]
            n92 = shared-variable ".\\Library 1.lvlib\\XYZ - rate_CIVITA [rad_s]"(w225) -> ()  [unwired: 1 in, 1 out]
          }
          frame Error {
            # "Error occurred \nreading Bytes at \nSerial Port"
          }
        }
        n93 = Unbundle By Name(w217) -> ("status"=w223:bool)
        n94 = shared-variable ".\\Library 1.lvlib\\Stop_RT"() -> (w215:bool)  [unwired: 1 in, 1 out]
        n95 = Or(x=w223, y=w215) -> (x .or. y?=w216:bool)
        n96 = node-c288() -> ()  [unwired: 1 in, 1 out]
      }
      n97 = node-c288(w179) -> ()  [unwired: 1 out]
      n98 = VISA Close(VISA resource name=w160, error in (no error)=w161) -> (error out=w153:errorcluster)
      n99 = call <vilib>:"Simple Error Handler.vi"("error in (no error)"=w153) -> ()  [unwired: 1 in, 8 out]
      n100 = node-c288(w181) -> ()  [unwired: 1 out]
      n101 = VISA Close(VISA resource name=w167, error in (no error)=w166) -> (error out=w175:errorcluster)
      n102 = call <vilib>:"Simple Error Handler.vi"("error in (no error)"=w175) -> ()  [unwired: 1 in, 8 out]
    }
  }
  n103 = case shown="True" w14 {
    tunnel: w22 -> [_ w257]
    frame False {
    }
    frame True {
      (unwired) u32 921600  # baud rate
      w263 = u32 10000  # timeout (ms)
      w266 = u16 0 items=["None"=0, "XON/XOFF"=1, "RTS/CTS"=2, "DTR/DSR"=4]  # flow control
      w262 = u16 10 items=["1.0"=10, "1.5"=15, "2.0"=20]  # stop bits
      w261 = u16 0 items=["None", "Odd", "Even", "Mark", "Space"]  # parity
      w264 = FALSE  # End read on termination character?
      w265 = u8 10  # termination char (0xA = '\n' = LF)
      w267 = u16 8  # data bits
      w258 = u32 460800  # baud rate
      w259 = refnum<visa-resource-name> "COM4"  # VISA resource name
      # "TVA (E-BOX) Serial Communication"
      # "Close session to port."
      n104 = call-poly "VISA Configure Serial Port"("VISA resource name"=w259, "timeout (10sec)"=w263, "termination char\n(0xA = '\\n' = LF)"=w265, "Enable Termination\nChar (T)"=w264, "baud rate (9600)"=w258, "data bits (8)"=w267, "parity (0:none)"=w261, "error in (no error)"=w257, "stop bits (10: 1 bit)"=w262, "flow control (0:none)"=w266) -> ("VISA resource name out"=w270:refnum<visa-resource-name>, "error out"=w271:errorcluster)  [unwired: 4 out]
      n105 = node-c288() -> (w273:T5)  [unwired: 4 in]
      n106 = timed-loop {
        tunnel: w271 -> [w278]
        tunnel: w270 -> [w279]
        tunnel: [w277] -> w268
        tunnel: [w276] -> w269
        timing: w273 -> [_]
        timing-out: [_] -> w272
        stop <- w275 stop-if-true
        # "Read the bytes in the buffer."
        # "TVA data from Controler - True\nTVA data from TVA system - False"
        # "TVA only read timed loop"
        n107 = node-c288() -> ()  [unwired: 1 in, 1 out]
        n108 = while {
          tunnel: w279 -> [w292]
          tunnel: w278 -> [w291]
          tunnel: [w290] -> w281
          tunnel: [w289] -> w280
          stop <- w284 stop-if-true
          w293 = u32 2  # bytes to read
          n109 = shared-variable ".\\Library 1.lvlib\\Stop_RT"() -> (w286:bool)  [unwired: 1 in, 1 out]
          n110 = VISA Read(VISA resource name=w292, byte count=w293, error in (no error)=w291) -> (VISA resource name out=w290:refnum<visa-resource-name>, read buffer=w288:string, error out=w289:errorcluster)  [unwired: 1 out]
          "TVA sync bytes" <- w288
          n111 = Equal?(x=w288, y="ë") -> (x = y?=w285:bool)
          n112 = Or(x=w285, y=w286) -> (x .or. y?=w284:bool)
        }
        n113 = case shown="True" FALSE ("TVA Protocol") {
          tunnel: w280 -> [w298 w324]
          tunnel: w281 -> [w299 w323]
          tunnel: [w296 w326] -> w276
          tunnel: [w297 w325] -> w277
          frame False {
            # "TVA to Board Computer"
            n114 = case "Read bytes from port." shown="No Error" w298 {
              selector: w298 -> [w316 w321]
              tunnel: [w319 w321] -> w296
              tunnel: [w320 w322] -> w297
              tunnel: w299 -> [w317 w322]
              frame No Error {
                w318 = u32 85  # bytes to read
                n115 = VISA Read(VISA resource name=w317, byte count=w318, error in (no error)=w316) -> (VISA resource name out=w320:refnum<visa-resource-name>, read buffer=w314:string, return count=→"TVA bytes read 2":u32, error out=w319:errorcluster)
                "TVA string 2" <- w314
                n116 = String To Byte Array(string=w314) -> (unsigned byte array=w313:u8[])
                n117 = Insert Into Array(array=w313, index=0, new element #1=u8 235 ("new element/subarray"), new element #2=u8 144 ("new element/subarray")) -> (w312:u8[])
                n118 = call "RT_TVA_2_boardcomp_DATA_vPXI.vi"("TVA data"=w312) -> ("TVA_Yaw [deg]"=w301:dbl, "TVA_Pitch [deg]"=w302:dbl, "Act 315 Angle \"Yaw\""=w304:dbl, "Act 225 Angle \"Pitch\""=w305:dbl, "CRC Check over Byte #10 to byte #84"=→"CRC Check over Byte #10 to byte #84":bool, "Control Variables (extra variables)"=w306:dbl[], "CRC Check over Byte #2 to Byte #7"=→"CRC Check over Byte #2 to Byte #7 TVA2BComp":bool)  [unwired: 4 in]
                "ACT 225 Angle \"Pitch\"" <- w305
                "ACT 315 Angle \"Yaw\"" <- w304
                "Control Variables\n (extra variables)" <- w306
                n119 = Build Array(w304, w305) -> (w303:dbl[])
                n120 = Build Array(w302, w301) -> (w300:dbl[])
                n121 = shared-variable ".\\Library 1.lvlib\\Control Variables"(w306) -> ()  [unwired: 1 in, 1 out]
                n122 = shared-variable ".\\Library 1.lvlib\\Act_b_TVA"(w303) -> ()  [unwired: 1 in, 1 out]
                n123 = shared-variable ".\\Library 1.lvlib\\TVA"(w300) -> ()  [unwired: 1 in, 1 out]
              }
              frame Error {
                # "Error occurred \nreading Bytes at \nSerial Port"
              }
            }
          }
          frame True {
            # "Board Computer to TVA"
            n124 = case "Read bytes from port." shown="No Error" w324 {
              selector: w324 -> [w341 w346]
              tunnel: [w344 w346] -> w326
              tunnel: [w345 w347] -> w325
              tunnel: w323 -> [w342 w347]
              frame No Error {
                w343 = u32 30  # bytes to read
                # "Roll Rate angle: \nDMARS info for \nTVA simulation"
                n125 = VISA Read(VISA resource name=w342, byte count=w343, error in (no error)=w341) -> (VISA resource name out=w345:refnum<visa-resource-name>, read buffer=w339:string, return count=→"TVA bytes read":u32, error out=w344:errorcluster)
                "TVA string" <- w339
                n126 = String To Byte Array(string=w339) -> (unsigned byte array=w338:u8[])
                n127 = Insert Into Array(array=w338, index=0, new element #1=u8 235 ("new element/subarray"), new element #2=u8 144 ("new element/subarray")) -> (w337:u8[])
                n128 = call "RT_TVA_DATA_vPXI.vi"("TVA data"=w337) -> ("Roll Rate/angle"=w327:dbl[], "Yaw Angle"=w332:dbl, "Pitch Angle"=w333:dbl, "CRC Check over Byte #10 to byte #29"=→"CRC Check over Byte #10 to byte #29":bool, "Control Variables (extra variables)"=w328:dbl[], "CRC Check over Byte #2 to Byte #7"=→"CRC Check over Byte #2 to Byte #7":bool)  [unwired: 5 in]
                "Roll Rate/angle" <- w327
                "Control Variables (extra variables)" <- w328
                n129 = shared-variable ".\\Library 1.lvlib\\Control Variables"(w328) -> ()  [unwired: 1 in, 1 out]
                n130 = Build Array(w333, w332) -> (w331:dbl[])
                n131 = shared-variable ".\\Library 1.lvlib\\TVA"(w331) -> ()  [unwired: 1 in, 1 out]
                n132 = shared-variable ".\\Library 1.lvlib\\Roll Rate_angle"(w327) -> ()  [unwired: 1 in, 1 out]
              }
              frame Error {
                # "Error occurred \nreading Bytes at \nSerial Port"
              }
            }
          }
        }
        n133 = Unbundle By Name(w276) -> ("status"=w282:bool)
        n134 = shared-variable ".\\Library 1.lvlib\\Stop_RT"() -> (w274:bool)  [unwired: 1 in, 1 out]
        n135 = node-c288() -> ()  [unwired: 1 in, 1 out]
        n136 = Or(x=w282, y=w274) -> (x .or. y?=w275:bool)
      }
      n137 = node-c288(w272) -> ()  [unwired: 1 out]
      n138 = VISA Close(VISA resource name=w268, error in (no error)=w269) -> (error out=w260:errorcluster)
      n139 = call <vilib>:"Simple Error Handler.vi"("error in (no error)"=w260) -> ()  [unwired: 1 in, 8 out]
    }
  }
  n140 = String To Path(string="C:\\ni-rt\\2018.12.04_VS50_alcantara_5ms.csv") -> (path=w23:path)
  n141 = disable-structure shown="Enabled" {
    disable-tunnel: "," ("delimiter (\\t)") -> [w353 w355]
    disable-tunnel: "%.9f" ("format (%.3f)") -> [w352 w356]
    disable-tunnel: [w351 w354] -> w40
    disable-tunnel: w23 -> [w350 w357]
    frame Disabled {
      n142 = call-poly <vilib>:"Read From Spreadsheet File.vi"("delimiter (\\t)"=w353, "format (%.3f)"=w352, "file path (dialog if empty)"=w350) -> ("all rows"=w351:dbl[][])  [unwired: 4 in, 4 out]
    }
    frame Enabled {
      n143 = call-poly <vilib>:"Read Delimited Spreadsheet.vi"("file path (dialog if empty)"=w357, "format (%.3f)"=w356, "delimiter (\\t)"=w355) -> ("all rows"=w354:dbl[][])  [unwired: 7 in, 5 out]
    }
  }
  "all rows" <- w40
  n144 = Unbundle By Name(w4) -> ("Fe gain"=w10:dbl, "Cnalpha gain"=w9:dbl, "clp gain"=w8:dbl, "cld gain"=w7:dbl, "cmq gain"=w6:dbl, "cnr gain"=w5:dbl)
  n145 = Unbundle By Name(w1) -> ("Initial Euler Angles [deg]"=w20:dbl[])
  n146 = Index Array(array=w40, index (col) #1=w41, index (col) #2=w36, index (col) #3=w33, index (col) #4=w29, index (col) #5=w28, index (col) #6=w27) -> (element #1=w43:dbl[], element #2=w38:dbl[], element #3=w35:dbl[], element #4=w31:dbl[], element #5=w30:dbl[], element #6=w32:dbl[])  [unwired: 6 in]
  n147 = Index Array(array=w20, index #1=0 ("index")) -> (element #1=w18:dbl, element #2=w16:dbl, element #3=w17:dbl)  [unwired: 2 in]
  n148 = Multiply(x=w30, y=w6) -> (x*y=w25:dbl[])
  n149 = Multiply(x=w32, y=w5) -> (x*y=w24:dbl[])
  n150 = Multiply(x=w31, y=w7) -> (x*y=w26:dbl[])
  n151 = Multiply(x=w35, y=w8) -> (x*y=w34:dbl[])
  n152 = Multiply(x=w38, y=w9) -> (x*y=w37:dbl[])
  n153 = Multiply(x=w43, y=w10) -> (x*y=w42:dbl[])
  n154 = Bundle By Name(cluster=cluster{"phi":dbl, "theta":dbl, "psi":dbl} {"phi"=1.532, "theta"=1.286, "psi"=0.0} ("Initial Euler Angles [deg]"), "phi"=w18, "theta"=w16, "psi"=w17) -> (w3:cluster{"phi":dbl, "theta":dbl, "psi":dbl})
  n155 = shared-variable ".\\Library 1.lvlib\\Initial Euler Angles [deg]"(w3) -> ()  [unwired: 1 in, 1 out]
  n156 = Replace Array Subset(array=w40, new element #1=w42, index (col) #1=w41, new element #2=w37, index (col) #2=w36, new element #3=w34, index (col) #3=w33, new element #4=w26, index (col) #4=w29, new element #5=w25, index (col) #5=w28, new element #6=w24, index (col) #6=w27) -> (w39:dbl[][])  [unwired: 6 in]
  n157 = expression code="(x/180.0)*pi" "degrees to radians"(w3) -> (w2:cluster{"phi":dbl, "theta":dbl, "psi":dbl})
  n158 = node-c288() -> (w49:T5)  [unwired: 4 in]
  n159 = timed-loop {
    timing: w49 -> [_]
    timing-out: [_] -> w48
    tunnel: w39 -> [w427]
    tunnel: w45 -> [w453]
    tunnel: w22 -> [_]
    tunnel: w2 -> [w366]
    tunnel: w1 -> [w380]
    tunnel: w4 -> [w378]
    i -> [w440]
    stop <- w361 stop-if-true
    w395 = FALSE  # DMARS from TVA comm
    w450 = TRUE  # Pred?
    w518 = T12 0 items=["X-Y-Z", "X-Z-Y", "Y-X-Z", "Y-Z-X", "Z-X-Y", "Z-Y-X", "X-Y-X", "X-Z-X", "Y-X-Y", "Y-Z-Y", "Z-X-Z", "Z-Y-Z"] ("rotation order")
    # "Rocket Dynamics"
    # "TVA"
    # "Euler Angles to table"
    # "Integration"
    # "INS"
    # "ATIVAR QUANDO HOUSEKEEPING DATA É USADO"
    # "DEG"
    # "TVA plant predictor and\ninertial to body"
    # "True = Civita info\nfalse = sim info"
    # "0 - Constant values\n1 - Received TVA cmds\n2 - Simulated control"
    # "Control"
    # "DMARS data"
    # "Rotation integration"
    # "Translation integration"
    # "Time"
    # "Vehicle parameters"
    n160 = node-c288() -> (w493:i64, w524:i64)  [unwired: 1 in]
    "Iteration Duration [us]" <- w493
    n161 = Unbundle By Name(w380) -> ("Sim_Time [s]"=w379:dbl)
    "Sim_Time [s]" <- w379
    n162 = Unbundle By Name(w380) -> ("Control Selection"=w358:enum16{"Constant", "TVA E-BOX", "Sim Control"}, "CFN-61G Enable"=w381:bool)
    n163 = disable-structure shown="Enabled" {
      disable-tunnel: ["Run_SIMULATION" w528] -> w512
      disable-tunnel: ["stop RT" w527] -> w503
      frame Disabled {
      }
      frame Enabled {
        n164 = shared-variable "NI-PXI8106\\Library 1.lvlib\\Stop_SIM"() -> (w527:bool)  [unwired: 1 in, 1 out]
        n165 = shared-variable "NI-PXI8106\\Library 1.lvlib\\Run_SIM"() -> (w528:bool)  [unwired: 1 in, 1 out]
      }
    }
    n166 = Greater?(x=w493, y=i64 10000) -> (0:→"bad iteration":bool)
    n167 = Unbundle By Name(w380) -> ("CFN-61G Enable"=w382:bool)
    n168 = call "Time (SubVI).vi"("Period"=w524, "Sim_Time [s]"=w379, "stop RT"=w503, "Run_SIMULATION"=w512) -> ("Stop"=w361:bool, "SIM_Running"=→"SIM_Running":bool, "i, sim_running, t[s], dt[s]"=w373:T13, "Sim t [s]"=→"Current time [s]":dbl)  [unwired: 4 in]
    n169 = Unbundle By Name(w373) -> ("sim_running"=w416:bool)
    n170 = shared-variable ".\\Library 1.lvlib\\Euler Angles_CIVITA"() -> (w490:sgl[])  [unwired: 1 in, 1 out]
    n171 = shared-variable ".\\Library 1.lvlib\\XYZ - rate_CIVITA [rad_s]"() -> (w488:sgl[])  [unwired: 1 in, 1 out]
    n172 = shared-variable ".\\Library 1.lvlib\\Stop_RT"(w361) -> ()  [unwired: 1 in, 1 out]
    n173 = Unbundle By Name(w373) -> ("sim_running"=w462:bool, "t[s]"=w461:dbl)
    n174 = Not(x=w416) -> (.not. x?=w414:bool)
    n175 = call "CIVITA_DMARS_conv_PXI(SubVI).vi"("Initial Euler Angles [rad]"=w366, "SIM_start"=w414, "Civitanav readings [deg]"=w490) -> ("Euler Angles [rad]"=w392:cluster{"phi":dbl, "theta":dbl, "psi":dbl})  [unwired: 5 in, 3 out]
    n176 = Index Array(array=w488, index #1=0 ("index")) -> (element #1=w486:sgl, element #2=w484:sgl, element #3=w485:sgl)  [unwired: 2 in]
    n177 = expression code="(x/pi)*180.0" "radians to degrees"(w392) -> (→"CIVITA as DMARS [º]":cluster{"phi":dbl, "theta":dbl, "psi":dbl})
    n178 = call "Euler_ang2quat RAD(SubVI).vi"("Euler Angles [rad]"=w392) -> ("Quaternions"=w489:dbl[])  [unwired: 10 in]
    n179 = Negate(x=w484) -> (-x=w483:sgl)
    n180 = Build Array(w485, w483, w486) -> (w482:sgl[])
    n181 = To Double Precision Float(number=w482) -> (double precision float=w481:dbl[])
    n182 = shared-variable ".\\Library 1.lvlib\\Roll Rate_angle"() -> (w399:dbl[])  [unwired: 1 in, 1 out]
    n183 = call "roll rate_angle(SubVI).vi"("Roll Rate/angle [deg]"=w399) -> ("Roll Angle[rad]"=w397:dbl[], "Roll Rate[rad/s]"=w398:dbl[])  [unwired: 9 in]
    n184 = Not(x=w462) -> (.not. x?=w415:bool)
    n185 = Build Array(w398, w397) -> (w396:dbl[][])
    n186 = shared-variable ".\\Library 1.lvlib\\Act_b_TVA"() -> (w385:dbl[])  [unwired: 1 in, 1 out]
    n187 = feedback #1(dbl[] [0.0, 0.0] ("TVA_cmd")) -> (w478:dbl[])
    n188 = case shown="True" TRUE {
      tunnel: [w563 w566] -> w444
      tunnel: w478 -> [w563 w564]
      tunnel: w415 -> [_ w565]
      frame False {
      }
      frame True {
        # "TVA plant"
        n189 = call "RT_Act_Plant_5ms_2_v1 (SubVI).vi"("not.Sim_Running"=w565, "TVA_cmd"=w564) -> ("Act_b"=w566:dbl[])  [unwired: 7 in, 2 out]
      }
    }
    n190 = expression code="(x/180.0)*pi" ("degrees to radians")(w385) -> (w441:dbl[])
    n191 = Select(t=w441, s=FALSE, f=w444) -> (s? t:f=w386:dbl[])
    n192 = shared-variable ".\\Library 1.lvlib\\Act_b_rad"(w444) -> ()  [unwired: 1 in, 1 out]
    n193 = call "Oil_Consumption (SubVI).vi"("act_b"=w386, "not.Sim_Running"=w415) -> ("Oil Consumption [L]"=w383:dbl)  [unwired: 9 in]
    n194 = Unbundle By Name(w378) -> ("dl [º]"=w377:dbl, "Nozzle misalignment yaw/pitch [º]"=w376:dbl[], "Nozzle eccentricity x/y [m]"=w375:dbl[])
    n195 = Bundle By Name(cluster=T8 {"act_b [rad]"=[], "Oil Consumption [L]"=0.0, "Act_b_TVA (315,225) [deg]"=[]} ("TVA"), "act_b [rad]"=w386, "Oil Consumption [L]"=w383, "Act_b_TVA (315,225) [deg]"=w385) -> (w384:T8)
    n196 = call "Vehicle Parameters (SubVI).vi"("Nozzle eccentricity x/y [m] in"=w375, "Nozzle misalignment yaw/pitch [º] in"=w376, "dl [º]"=w377) -> ("Vehicle Parameters"=w436:T14)  [unwired: 8 in]
    n197 = expression code="(x/pi)*180.0" "radians to degrees"(w366) -> (w365:cluster{"phi":dbl, "theta":dbl, "psi":dbl})
    n198 = Unbundle By Name(w380) -> ("V_ini [m/s]"=w412:dbl[], "latd_ini [º]"=w411:dbl, "lon_ini [º]"=w410:dbl, "altitude_ini(m)"=w409:dbl)
    n199 = Unbundle By Name(w380) -> ("W_b ini [rad/s]"=w408:dbl[], "W ini [rad/s]"=w407:dbl[])
    n200 = Unbundle By Name(w373) -> ("dt [s]"=w363:dbl, "sim_running"=w423:bool)
    n201 = Unbundle By Name(w373) -> ("t[s]"=w359:dbl, "sim_running"=w374:bool)
    n202 = call "Euler_ang2quat(SubVI).vi"("Euler Angles [deg]"=w365) -> ("Quaternions"=w449:dbl[])  [unwired: 10 in]
    n203 = Not(x=w423) -> (.not. x?=w424:bool)
    n204 = expression code="(x/180.0)*pi" "degrees to radians"(w411) -> (w510:dbl)
    n205 = expression code="(x/180.0)*pi" "degrees to radians"(w410) -> (w507:dbl)
    n206 = feedback #2(w408) -> (w505:dbl[])
    n207 = Select(t=w408, s=w424, f=w505) -> (s? t:f=w445:dbl[])
    n208 = feedback #3(w407) -> (w497:dbl[])
    n209 = Select(t=w407, s=w424, f=w497) -> (s? t:f=w471:dbl[])
    n210 = feedback #4(w449) -> (w504:dbl[])
    n211 = Select(t=w449, s=w424, f=w504) -> (s? t:f=w455:dbl[])
    n212 = call "RT_q2DCM (SubVI).vi"("Quaternion"=w455) -> ("DCM"=w454:dbl[][])  [unwired: 10 in]
    n213 = call "Sub_predictor_v4(SubVI).vi"("predicted step"="predicted step", "Sim_running"=w374, "q_i"=w455, "Pred ?"=w450, "t [s]"=w359) -> ("Euler Angles Table_pred [deg]"=w491:dbl[], "DMARS SIM pred [º]"=→"DMARS SIM pred[º]":cluster{"phi":dbl, "theta":dbl, "psi":dbl})  [unwired: 3 in, 2 out]
    "Table cmd [º] inner middle outer" <- w491
    n214 = call <vilib>:"Direction Cosines To Euler Angles.vi"("rotation order"=w518, "Direction Cosines"=w454) -> ("Euler Angles"=w515:cluster{"phi":dbl, "theta":dbl, "psi":dbl})  [unwired: 8 in, 1 out]
    n215 = shared-variable ".\\Library 1.lvlib\\Euler Angles Table [deg]"(w491) -> ()  [unwired: 1 in, 1 out]
    n216 = Unbundle(w515) -> ("phi"=w517:dbl, "theta"=w516:dbl, "psi"=w514:dbl)
    n217 = feedback #5(w412) -> (w509:dbl[])
    n218 = Select(t=w412, s=w424, f=w509) -> (s? t:f=w460:dbl[])
    n219 = feedback #6(w510) -> (w511:dbl)
    n220 = Select(t=w510, s=w424, f=w511) -> (s? t:f=w446:dbl)
    n221 = feedback #7(w507) -> (w508:dbl)
    n222 = Select(t=w507, s=w424, f=w508) -> (s? t:f=w447:dbl)
    n223 = feedback #8(w409) -> (w506:dbl)
    n224 = Select(t=w409, s=w424, f=w506) -> (s? t:f=w463:dbl)
    n225 = Build Array(w517, w516, w514) -> (w364:dbl[])
    n226 = Bundle By Name ("importante para o inicio")(cluster="Rotation", "W_b(i) [rad/s]"=w445, "W(i) [rad/s]"=w471, "q(i)"=w455, "Euler Angles {rad]"=w364) -> (w418:T3)
    n227 = Unbundle By Name(w418) -> ("W_b(i) [rad/s]"=w389:dbl[], "q(i)"=w417:dbl[])
    n228 = Unbundle By Name(w418) -> ("q(i)"=w429:dbl[])
    n229 = call "RT_q2DCM (SubVI).vi"("Quaternion"=w429) -> ("DCM"=w430:dbl[][])  [unwired: 10 in]
    n230 = call-poly <vilib>:"Array To Matrix.vi"("Real 2D Array"=w430) -> ("Real Matrix"=w431:T15)
    n231 = Select(t=w489, s=w382, f=w417) -> (s? t:f=w368:dbl[])
    n232 = Select(t=w481, s=w382, f=w389) -> (s? t:f=w393:dbl[])
    n233 = call "quat2eulerXYZ.vi"("Quaternions"=w368) -> ("Euler Angles [rad]"=w367:cluster{"phi":dbl, "theta":dbl, "psi":dbl})  [unwired: 10 in]
    n234 = Unbundle(w367) -> ("phi"=w372:dbl, "theta"=w371:dbl, "psi"=w370:dbl)
    n235 = Build Array(w372, w371, w370) -> (w369:dbl[])
    n236 = Build Array(w393, w369) -> (w394:dbl[][])
    n237 = Select(t=w396, s=w395, f=w394) -> (s? t:f=w388:dbl[][])
    n238 = Index Array(array=w388) -> (element #1=w391:dbl[], element #2=w390:dbl[])  [unwired: 4 in]
    n239 = Index Array(array=w390, index=2) -> (element=w451:dbl)
    n240 = call "RT_TVAr_i (SubVI).vi"("roll1"=w451, "Act315_Act225"=w441) -> ("TVA_p/TVA_y"=w442:dbl[])  [unwired: 13 in]
    n241 = expression code="(x/pi)*180.0" ("radians to degrees")(w442) -> (w475:dbl[])
    n242 = shared-variable ".\\Library 1.lvlib\\TVA_p_TVA_y_rec"(w475) -> ()  [unwired: 1 in, 1 out]
    n243 = disable-structure shown="Disabled" {
      frame Disabled {
        (unwired) dbl[] [0.9999619154929337, 0.006684456018117924, 0.0056110787342547866, 3.750843750367606e-05]  # [0.766 - 0.643 - 0]
        (unwired) dbl[] [0.9996567767353742, 0.020067092257636514, 0.016838238751872656, 0.00033801050355844806]  # [2.3 - 1.93 - 0]
        # "Quats de atitudes iniciais"
      }
      frame Enabled {
      }
    }
    n244 = Bundle By Name ("importante para o inicio")(cluster=T11 {"latd(i) [rad]"=0.0, "lon(i) [rad]"=0.0, "height(i)(m)"=0.0, "V(i) [m/s] NWU"=[]} ("Position"), "V(i) [m/s] NWU"=w460, "latd(i) [rad]"=w446, "lon(i) [rad]"=w447, "height(i)(m)"=w463) -> (w422:T11)
    n245 = Unbundle By Name(w422) -> ("latd(i) [rad]"=w421:dbl, "lon(i) [rad]"=w420:dbl, "height(i)(m)"=w419:dbl, "V(i) [m/s] NWU"=w401:dbl[])
    n246 = Index Array(array=w401, index #1=0 ("index")) -> (element #1=w403:dbl, element #2=w405:dbl, element #3=w402:dbl)  [unwired: 2 in]
    n247 = Negate(x=w405) -> (-x=w404:dbl)
    n248 = Build Array(w403, w404, w402) -> (w400:dbl[])
    n249 = Build Array(w421, w420, w419) -> (w498:dbl[])
    n250 = call "Rocket Dynamics (SubVI).vi"("Rotation"=w418, "Position"=w422, "Time"=w373, "TVA"=w384, "Vehicle Param"=w436, "V_Wind [m/s]"=w453, "Data"=w427) -> ("Aerodyn output"=w426:T16, "ang_acc"=w362:dbl[], "M_alpha [rad/s^2], M_beta [rad/s^2]"=w425:T17, "acc [m/s^2]"=w360:dbl[])  [unwired: 1 in]
    n251 = call-poly <vilib>:"Array To Matrix.vi"("Real 1D Array"=w360) -> ("Real Matrix (Column Vector)"=w432:T15)
    n252 = call-poly <vilib>:"A x B.vi"("B"=w432, "A"=w431) -> ("A x B"=w434:T15)  [unwired: 1 out]
    n253 = call-poly <vilib>:"Matrix To Array.vi"("Real Matrix"=w434) -> ("Real 2D Array"=w433:dbl[][])
    n254 = Index Array "acc_b"(array=w433, index (col)=0 ("index (row)")) -> (element=w428:dbl[])  [unwired: 1 in]
    n255 = Insert Into Array(array=dbl[] [], index=0, new element #1=w393, new element #2=w428, new element #3=w368, new element #4=w400, new element #5=w498) -> (w494:dbl[])
    n256 = disable-structure shown="Enabled" {
      disable-tunnel: w494 -> [w561 w562]
      disable-tunnel: w416 -> [w530 _]
      disable-tunnel: [w529 w562] -> w479
      frame Disabled {
        w542 = dbl[] [0.0, 0.0, 0.0, 0.0, 0.0, 0.0, 0.0, 0.0, 0.0, 0.0, 0.0, 0.0, 0.0, 0.0, 0.0, 0.0] ("TVA_cmd")
        w544 = dbl[] [0.0, 0.0, 0.0, 0.0, 0.0, 0.0, 0.0, 0.0, 0.0, 0.0, 0.0, 0.0, 0.0, 0.0, 0.0, 0.0] ("TVA_cmd")
        w545 = dbl[] [0.0, 0.0, 0.0, 0.0, 0.0, 0.0, 0.0, 0.0, 0.0, 0.0, 0.0, 0.0, 0.0, 0.0, 0.0, 0.0] ("TVA_cmd")
        w546 = dbl[] [0.0, 0.0, 0.0, 0.0, 0.0, 0.0, 0.0, 0.0, 0.0, 0.0, 0.0, 0.0, 0.0, 0.0, 0.0, 0.0] ("TVA_cmd")
        w547 = dbl[] [0.0, 0.0, 0.0, 0.0, 0.0, 0.0, 0.0, 0.0, 0.0, 0.0, 0.0, 0.0, 0.0, 0.0, 0.0, 0.0] ("TVA_cmd")
        w553 = dbl[] [0.0, 0.0, 0.0, 0.0, 0.0, 0.0, 0.0, 0.0, 0.0, 0.0, 0.0, 0.0, 0.0, 0.0, 0.0, 0.0] ("TVA_cmd")
        w555 = dbl[] [0.0, 0.0, 0.0, 0.0, 0.0, 0.0, 0.0, 0.0, 0.0, 0.0, 0.0, 0.0, 0.0, 0.0, 0.0, 0.0] ("TVA_cmd")
        w557 = dbl[] [0.0, 0.0, 0.0, 0.0, 0.0, 0.0, 0.0, 0.0, 0.0, 0.0, 0.0, 0.0, 0.0, 0.0, 0.0, 0.0] ("TVA_cmd")
        w559 = dbl[] [0.0, 0.0, 0.0, 0.0, 0.0, 0.0, 0.0, 0.0, 0.0, 0.0, 0.0, 0.0, 0.0, 0.0, 0.0, 0.0] ("TVA_cmd")
        w556 = dbl[] [0.0, 0.0, 0.0, 0.0, 0.0, 0.0, 0.0, 0.0, 0.0, 0.0, 0.0, 0.0, 0.0, 0.0, 0.0, 0.0] ("TVA_b")
        # "Simulated DMARS"
        n257 = feedback #9(w559) -> (w560:dbl[])
        n258 = Select(t=w559, s=w530, f=w560) -> (s? t:f=w552:dbl[])
        n259 = feedback-in #9(w561) -> ()
        n260 = feedback #10(w557) -> (w558:dbl[])
        n261 = Select(t=w557, s=w530, f=w558) -> (s? t:f=w551:dbl[])
        n262 = feedback-in #10(w552) -> ()
        n263 = feedback #11(w555) -> (w541:dbl[])
        n264 = Select(t=w555, s=w530, f=w541) -> (s? t:f=w536:dbl[])
        n265 = feedback-in #11(w551) -> ()
        n266 = feedback #12(w547) -> (w540:dbl[])
        n267 = Select(t=w547, s=w530, f=w540) -> (s? t:f=w535:dbl[])
        n268 = feedback-in #12(w536) -> ()
        n269 = feedback #13(w546) -> (w539:dbl[])
        n270 = Select(t=w546, s=w530, f=w539) -> (s? t:f=w534:dbl[])
        n271 = feedback-in #13(w535) -> ()
        n272 = feedback #14(w545) -> (w538:dbl[])
        n273 = Select(t=w545, s=w530, f=w538) -> (s? t:f=w533:dbl[])
        n274 = feedback-in #14(w534) -> ()
        n275 = feedback #15(w544) -> (w537:dbl[])
        n276 = Select(t=w544, s=w530, f=w537) -> (s? t:f=w531:dbl[])
        n277 = feedback-in #15(w533) -> ()
        n278 = feedback #16(w542) -> (w543:dbl[])
        n279 = Select(t=w542, s=w530, f=w543) -> (s? t:f=w532:dbl[])
        n280 = feedback-in #16(w531) -> ()
        n281 = feedback #17(w553) -> (w554:dbl[])
        n282 = Select(t=w553, s=w530, f=w554) -> (s? t:f=w550:dbl[])
        n283 = feedback #18(w556) -> (w548:dbl[])
        n284 = Select(t=w556, s=w530, f=w548) -> (s? t:f=w549:dbl[])
        n285 = call "RT_DMARS (SubVI).vi"("y2"=w549, "y1"=w550, "u8"=w532, "u7"=w531) -> ("DMARS Data"=w529:dbl[])  [unwired: 7 in]
        n286 = feedback-in #17(w529) -> ()
        n287 = feedback-in #18(w550) -> ()
      }
      frame Enabled {
      }
    }
    n288 = shared-variable ".\\Library 1.lvlib\\DMARS"(w479) -> ()  [unwired: 1 in, 1 out]
    n289 = call "RT_Rotation_Integration_v2 (SubVI).vi"("W_b(i) [rad/s]"=w445, "ang_acc [rad/s^2]"=w362, "q(i) in"=w455, "dt"=w363) -> ("W(i+1)"=w467:dbl[], "W_b(i+1) [rad/s]"=w466:dbl[], "q(i+1)"=w465:dbl[], "Euler angles (i+1) XYZ [rad]"=w464:dbl[])  [unwired: 12 in]
    n290 = feedback-in #2(w466) -> ()
    n291 = feedback-in #3(w467) -> ()
    n292 = feedback-in #4(w465) -> ()
    n293 = call "Translation_Integration2.vi"("acc"=w360, "V(i) in"=w460, "latd(i)"=w446, "lon(i) [rad]"=w447, "height(i) [m]"=w463, "dt [s]"=w363) -> ("position"=w513:dbl[], "position ECEF (i) [m]"=w473:dbl[], "Lat_C [rad]"=w472:dbl, "Velocity"=w459:dbl[])  [unwired: 10 in]
    n294 = feedback-in #5(w459) -> ()
    n295 = Bundle By Name(cluster=T9 {"W(i+1) [rad/s]"=[], "W_b(i+1) [rad/s]"=[], "q(i+1)"=[], "Euler angles (i+1) XYZ [rad]"=[]} ("output cluster 2"), "W(i+1) [rad/s]"=w467, "W_b(i+1) [rad/s]"=w466, "q(i+1)"=w465, "Euler angles (i+1) XYZ [rad]"=w464) -> (w452:T9)
    n296 = case shown="\"Sim Control\"" w358 {
      tunnel: [w568 w574 w604] -> w502
      tunnel: [w567 w575 w603] -> w501
      tunnel: [_ w581 _] -> w480
      tunnel: w427 -> [_ _ w599]
      tunnel: w461 -> [_ w573 w607]
      tunnel: w440 -> [_ _ w614]
      tunnel: w392 -> [_ _ w594]
      tunnel: w462 -> [_ w576 w596]
      tunnel: w452 -> [_ _ w601]
      tunnel: w422 -> [_ _ w602]
      tunnel: w425 -> [_ _ w600]
      tunnel: w373 -> [_ _ w598]
      tunnel: w418 -> [_ _ w597]
      tunnel: w381 -> [_ _ w593]
      frame "Constant", Default {
        w567 = 0.0  # Pitch
        w568 = 0.0  # Yaw
      }
      frame "TVA E-BOX" {
        w583 = T18 2 items=["1-norm"=1, "2-norm"=2, "Inf-norm"=3, "-Inf-norm"=4, "User Defined"=5] ("norm type")
        n297 = shared-variable ".\\Library 1.lvlib\\TVA"() -> (w570:dbl[])  [unwired: 1 in, 1 out]
        "TVA_cmd [deg] 2" <- w570
        n298 = call-poly <vilib>:"Vector Norm.vi"("norm type"=w583, "Input Vector"=w570) -> ("norm"=w569:dbl)  [unwired: 8 in, 1 out]
        n299 = Divide(x=w570, y=w569) -> (x/y=w578:dbl[])
        n300 = Greater?(x=w569, y=3.0) -> (0:w580:bool)
        n301 = Multiply(x=3.0 ("y"), y=w578) -> (x*y=w577:dbl[])
        n302 = Select(t=w577, s=w580, f=w570) -> (s? t:f=w581:dbl[])
        n303 = Index Array(array=w581, index #1=0 ("index")) -> (element #1=w572:dbl, element #2=w571:dbl)  [unwired: 1 in]
        n304 = disable-structure shown="Enabled" {
          disable-tunnel: w576 -> [w590 _]
          disable-tunnel: [w589 w592] -> w575
          disable-tunnel: [w588 w591] -> w574
          disable-tunnel: w573 -> [w587 _]
          disable-tunnel: w572 -> [w586 w592]
          disable-tunnel: w571 -> [w585 w591]
          frame Disabled {
            n305 = call "TVA_cmd_LMS(SubVI).vi"("t [s]"=w587, "Sim_running"=w590, "TVA_yaw"=w585, "TVA_pitch"=w586) -> ("TVA_yaw_LMS"=w588:dbl, "TVA_pitch_LMS"=w589:dbl)  [unwired: 6 in]
          }
          frame Enabled {
          }
        }
      }
      frame "Sim Control" {
        n306 = Quotient & Remainder(x=w614, y=2) -> (x-y*floor(x/y)=w612:i32)  [unwired: 1 out]
        n307 = Not Equal To 0?(x=w612) -> (x != 0?=w610:bool)
        n308 = call "Control_2.vi"("latd-lon-heig-VNWU"=w602, "CIVITA as DMARS [rad]"=w594, "Wi1-Wbi1-qi1-Euli1"=w601, "Civita?"=w593, "Mab"=w600, "File"=w599, "dt-sim_run-t-i"=w598, "Rotation"=w597, "sim_running"=w596) -> ("TVA_cmd(i+1,:) [deg]"=w595:dbl[])  [unwired: 4 in, 2 out]
        n309 = Index Array(array=w595, index #1=0 ("index")) -> (element #1=w611:dbl, element #2=w608:dbl)  [unwired: 1 in]
        n310 = case shown="False" FALSE {
          tunnel: [w625 w631] -> w606
          tunnel: [w624 w630] -> w605
          tunnel: w611 -> [w625 w629]
          tunnel: w608 -> [w624 w628]
          tunnel: w610 -> [_ w627]
          frame False {
          }
          frame True {
            # "10ms output"
            n311 = feedback #19(w629) -> (w626:dbl)
            n312 = feedback #20(w628) -> (w632:dbl)
            n313 = Select(t=w629, s=w627, f=w626) -> (s? t:f=w631:dbl)
            n314 = feedback-in #19(w631) -> ()
            n315 = Select(t=w628, s=w627, f=w632) -> (s? t:f=w630:dbl)
            n316 = feedback-in #20(w630) -> ()
          }
        }
        n317 = disable-structure shown="Enabled" {
          disable-tunnel: w596 -> [w621 _]
          disable-tunnel: w607 -> [w620 _]
          disable-tunnel: w606 -> [w619 w623]
          disable-tunnel: w605 -> [w618 w622]
          disable-tunnel: [w617 w623] -> w604
          disable-tunnel: [w616 w622] -> w603
          frame Disabled {
            n318 = call "TVA_cmd_LMS(SubVI).vi"("t [s]"=w620, "Sim_running"=w621, "TVA_yaw"=w618, "TVA_pitch"=w619) -> ("TVA_yaw_LMS"=w616:dbl, "TVA_pitch_LMS"=w617:dbl)  [unwired: 6 in]
          }
          frame Enabled {
          }
        }
      }
    }
    "TVA_cmd [deg]" <- w480
    n319 = expression code="(x/180.0)*pi" "degrees to radians"(w501) -> (w499:dbl)
    n320 = expression code="(x/180.0)*pi" "degrees to radians"(w502) -> (w500:dbl)
    n321 = Build Array(w500, w499) -> (w439:dbl[])
    n322 = call "Act_cmd_2 (SubVI).vi"("W_b [rad/s]"=w391, "Euler Angles [rad]"=w390, "TVA_cmd [rad]"=w439) -> ("Act315_Act225"=w477:dbl[])  [unwired: 7 in, 1 out]
    n323 = feedback-in #1(w477) -> ()
    n324 = Index Array(array=w513, index #1=0 ("index")) -> (element #1=w470:dbl, element #2=w469:dbl, element #3=w468:dbl)  [unwired: 2 in]
    n325 = feedback-in #6(w470) -> ()
    n326 = feedback-in #7(w469) -> ()
    n327 = feedback-in #8(w468) -> ()
    n328 = Bundle By Name(cluster=T10 {"position ECEF (i)"=[], "Lat_C [rad]"=0.0, "latd(i+1) [rad]"=0.0, "lon(i+1) [rad]"=0.0, "height (i+1) [m]"=0.0, "V(i+1) [m/s] NWU"=[]} ("output cluster 2"), "position ECEF (i)"=w473, "Lat_C [rad]"=w472, "latd(i+1) [rad]"=w470, "lon(i+1) [rad]"=w469, "height (i+1) [m]"=w468, "V(i+1) [m/s] NWU"=w459) -> ()  [unwired: 1 out]
    n329 = call "LOG_sim_2 (SubVI).vi"("Rotation"=w418, "Time"=w373, "act_b"=w384, "Position"=w422, "Aerodyn"=w426, "M_alpha [rad/s^2], M_beta [rad/s^2]"=w425, "acc [m/s^2]"=w360) -> ()  [unwired: 5 in]
    n330 = node-c288() -> ()  [unwired: 1 in, 1 out]
  }
  n331 = Unbundle By Name(w1) -> ("Table enable"=w12:bool)
  n332 = case shown="True" w12 {
    tunnel: w22 -> [_ _]
    frame False {
    }
    frame True {
      w642 = 10000 ("timeout ms (60000)")
      w658 = i64 5000  # Period [us]
      # "Motion Simulation Table control and LOG"
      n333 = disable-structure shown="Enabled" {
        disable-tunnel: [w679 w690] -> w659
        disable-tunnel: [w677 w688] -> w651
        frame Disabled {
          # "Path shown is for NI Linux RTOS\ntargets. VxWorks path is c:\\test1.txt"
          n334 = Get Date/Time In Seconds() -> (seconds since 1Jan1904=w670:timestamp)
          n335 = case shown="False" FALSE {
            tunnel: [".txt" ("string") ".csv" ("string")] -> w674
            frame False {
            }
            frame True {
            }
          }
          n336 = Format Date/Time String(time format string (%c)="%d%m%Y_%H%M%S", seconds (now)=w670, UTC format="UTC format") -> (date/time string=w669:string)
          n337 = Concatenate Strings(w669, w674) -> (w675:string)
          "concatenated string" <- w675
          n338 = Build Path(base path=path "c:/" ("file path (use dialog)"), name or relative path=w675) -> (appended path=w673:path)
          "appended path" <- w673
          n339 = Open/Create/Replace File(file path (use dialog)=w673, operation (0:open)=T19."replace or create") -> (refnum out=w677:refnum<file>, error out=w679:errorcluster)  [unwired: 4 in, 1 out]
        }
        frame Enabled {
          # "Path shown is for NI Linux RTOS\ntargets. VxWorks path is c:\\test1.txt"
          n340 = case shown="False" FALSE {
            tunnel: [".txt" ("string") ".csv" ("string")] -> w685
            frame False {
            }
            frame True {
            }
          }
          n341 = Concatenate Strings("LOG" ("time format string (%c)"), w685) -> (w686:string)
          "concatenated string 2" <- w686
          n342 = Build Path(base path=path "c:/" ("file path (use dialog)"), name or relative path=w686) -> (appended path=w684:path)
          "PXI log path 2" <- w684
          n343 = Open/Create/Replace File(file path (use dialog)=w684, operation (0:open)=T19."replace or create") -> (refnum out=w688:refnum<file>, error out=w690:errorcluster)  [unwired: 4 in, 1 out]
        }
      }
      n344 = shared-variable ".\\Library 1.lvlib\\Initial Euler Angles [deg]"() -> (w648:cluster{"phi":dbl, "theta":dbl, "psi":dbl})  [unwired: 1 in, 1 out]
      "Initial Euler Angles [deg] 2" <- w648
      n345 = UDP Open(9:w642, 11:u16 9838 ("port")) -> (port=w656:refnum<k16>, 0:w641:errorcluster)  [unwired: 1 in, 3 out]
      n346 = TCP Open Connection(address="Remote Host", remote port or service name=u16 9878, timeout ms (60000)=w642) -> (connection ID=w655:refnum<k5>, error out=w643:errorcluster)  [unwired: 2 in]
      n347 = String To IP(1:"Remote Host") -> (0:w657:u32)
      n348 = Merge Errors(w643, w641) -> (w646:errorcluster)
      n349 = call "Time Delay"("error in (no error)"=w646) -> ("error out"=w654:errorcluster)  [unwired: 10 in]
      n350 = call "Start_track.vi"("TCP connection ID"=w655, "UDP connection ID"=w656, "IP address in"=w657, "Euler Angles DMARS [º] debug"=w648, "error in"=w654) -> ("TCP connection ID out"=w660:refnum<k5>, "UDP connection ID out"=w664:refnum<k16>, "IP address out"=w663:u32, "error out"=w662:errorcluster)  [unwired: 6 in, 1 out]
      n351 = node-c288(w658) -> (w653:T5)  [unwired: 3 in]
      n352 = node-c288(w658) -> (w667:T5)  [unwired: 3 in]
      n353 = timed-loop {
        tunnel: w651 -> [w703]
        tunnel: [w702] -> w650
        timing: w653 -> [_]
        timing-out: [_] -> w652
        shift-right: [w697] -> w649
        shift-left: w659 -> [w698]
        stop <- w701 stop-if-true
        n354 = node-c288() -> ()  [unwired: 1 in, 1 out]
        n355 = shared-variable ".\\Library 1.lvlib\\Sim_logdata"() -> (w696:dbl[])  [unwired: 1 in, 1 out]
        n356 = shared-variable ".\\Library 1.lvlib\\output array"() -> (w695:dbl[])  [unwired: 1 in, 1 out]
        n357 = Insert Into Array(array=w696, index=34, new element=w695) -> (w693:dbl[])
        n358 = shared-variable ".\\Library 1.lvlib\\Stop_RT"() -> (w701:bool)  [unwired: 1 in, 1 out]
        n359 = Array To Spreadsheet String(array=w693, 3:"%g;" ("format string")) -> (spreadsheet string=w699:string)  [unwired: 1 in]
        "spreadsheet string" <- w699
        n360 = node-c288() -> ()  [unwired: 1 in, 1 out]
        n361 = Write to Text File(file (use dialog)=w703, text=w699, error in=w698) -> (refnum out=w702:refnum<file>, error out=w697:errorcluster)  [unwired: 1 in, 1 out]
      }
      n362 = timed-loop {
        timing: w667 -> [_]
        timing-out: [_] -> w666
        tunnel: w664 -> [w804]
        tunnel: w663 -> [w803]
        tunnel: w662 -> [w802]
        tunnel: [w806] -> w661
        tunnel: [w805] -> w665
        tunnel: w659 -> [_]
        stop <- w788 stop-if-true
        w712 = 0.0
        w711 = 0.0
        w710 = 0.0
        w713 = TRUE ("s")
        w720 = 10.0 ("x")
        w781 = 0
        # "Time"
        # "Guidance = F"
        # "Send and receive table data"
        # "True when simulation starts"
        # "predictor"
        # "Data for log file"
        # "time_motion table\ninner p cmd [deg]\ninner r cmd  [deg/s]\ninner a cmd  [deg/s^2]\nmiddle p cmd  [deg]\nmiddle r cmd  [deg/s]\nmiddle a cmd [deg/s^2]\nouter p cmd [deg]\nouter r cmd [deg/s]\nouter a cmd [deg/s^2]\ninner p mon [deg]\ninner r mon [deg/s]\ninner a mon [deg/s^2]\nmiddle p mon [deg]\nmiddle r mon [deg/s]\nmiddle a mon [deg/s^2]\nouter p mon [deg]\nouter r mon [deg/s]\nouter a mon [deg/s^2]\nTVA Pitch_rec [deg]\nTVA Yaw_rec [deg]\n-\nTVA_pitch_cmd [deg]\nTVA_yaw_cmd [deg]\nAct_pitch_from cmd [deg] / Distance ground\nAct_yaw_from cmd [deg] / Distance alt"
        # "34\n35\n36\n37\n38\n39\n40\n41\n42\n43\n44\n45\n46\n47\n48\n49\n50\n51\n52\n53\n54\n55\n56\n57\n58\n59"
        n363 = node-c288() -> (w769:i64, →"Iteration Duration":i64)  [unwired: 1 in]
        "Period" <- w769
        n364 = shared-variable ".\\Library 1.lvlib\\Euler Angles Table [deg]"() -> (w761:dbl[])  [unwired: 1 in, 1 out]
        n365 = shared-variable ".\\Library 1.lvlib\\SIM_Running"() -> (w763:bool)  [unwired: 1 in, 1 out]
        n366 = To Double Precision Float(number=w769) -> (double precision float=w770:dbl)
        n367 = Divide(x=w770, y=1000000.0) -> (x/y=w768:dbl)
        n368 = disable-structure shown="Enabled" {
          disable-tunnel: [-90.0 ("y") 0.0 ("y")] -> w760
          frame Disabled {
          }
          frame Enabled {
          }
        }
        n369 = feedback #21(w781) -> (w782:i32)
        n370 = Select(t=w782, s=w763, f=w781) -> (s? t:f=w779:i32)
        n371 = Index Array(array=w761, index #1=0 ("index")) -> (element #1=w747:dbl, element #2=w759:dbl, element #3=w745:dbl)  [unwired: 2 in]
        n372 = To Double Precision Float(number=w779) -> (double precision float=w767:dbl)
        n373 = Increment(x=w779) -> (x+1=w780:i32)
        n374 = feedback-in #21(w780) -> ()
        n375 = Multiply "t [s]"(x=w768, y=w767) -> (x*y=w734:dbl)
        "Time (s)" <- w734
        n376 = Add(x=w759, y=w760) -> (x+y=w746:dbl)
        n377 = Equal To 0?(x=w734) -> (x = 0?=→"Table Ready":bool)
        n378 = shared-variable ".\\Library 1.lvlib\\Stop_RT"() -> (w788:bool)  [unwired: 1 in, 1 out]
        n379 = Bundle("Numeric"=w747, w711, w711) -> (w744:cluster{"Numeric":dbl, dbl, dbl})  [unwired: 1 in]
        n380 = Bundle(w746, w710, w710) -> (w743:cluster{dbl, dbl, dbl})  [unwired: 1 in]
        n381 = Bundle("Numeric"=w745, w712, w712) -> (w742:cluster{"Numeric":dbl, dbl, dbl})  [unwired: 1 in]
        n382 = call "Send_Demand_controlword.vi"("UDP connection ID out"=w804, "Inner TRACK"=w744, "Middle TRACK"=w743, "Outer TRACK"=w742, "IP address in"=w803, "error in"=w802, "ReadOnly"=FALSE) -> ("UDP connection ID out"=w726:refnum<k16>, "concatenated string"=→"string enviada para acutrol":string, "error out"=w728:errorcluster)  [unwired: 5 in, 1 out]
        n383 = call "Receive_Monitor.vi"("UDP connection ID"=w726, "error out 2"=w728) -> ("UDP connection ID out"=w805:refnum<k16>, "MonitorBlock"=w793:dbl[], "error out"=w806:errorcluster)  [unwired: 11 in]
        n384 = shared-variable ".\\Library 1.lvlib\\TVA_p_TVA_y_rec"() -> (w733:dbl[])  [unwired: 1 in, 1 out]
        n385 = shared-variable ".\\Library 1.lvlib\\TVA"() -> (w740:dbl[])  [unwired: 1 in, 1 out]
        n386 = shared-variable ".\\Library 1.lvlib\\Act_b_rad"() -> (w731:dbl[])  [unwired: 1 in, 1 out]
        n387 = shared-variable ".\\Library 1.lvlib\\Roll Rate_angle"() -> (w723:dbl[])  [unwired: 1 in, 1 out]
        n388 = Index Array(array=w793, index #1=0 ("index"), index #2=3 ("index"), index #3=6 ("index"), index #4=1 ("index"), index #5=4 ("index"), index #6=7 ("index"), index #7=2 ("index"), index #8=5 ("index"), index #9=8 ("index")) -> (element #1=w737:dbl, element #2=w757:dbl, element #3=w758:dbl, element #4=w735:dbl, element #5=w755:dbl, element #6=w753:dbl, element #7=w756:dbl, element #8=w754:dbl, element #9=w778:dbl)
        n389 = Index Array(array=w740, index #1=0 ("index")) -> (element #1=w739:dbl, element #2=w738:dbl)  [unwired: 1 in]
        n390 = Index Array(array=w731, index #1=0 ("index")) -> (element #1=w730:dbl, element #2=w729:dbl)  [unwired: 1 in]
        n391 = Index Array(array=w723, index #1=0 ("index")) -> (element #1=w722:dbl, element #2=w721:dbl)  [unwired: 1 in]
        n392 = Unbundle(w744) -> ("Numeric"=w765:dbl, w777:dbl, w776:dbl)
        n393 = Unbundle(w743) -> (w764:dbl, w775:dbl, w774:dbl)
        n394 = Unbundle(w742) -> ("Numeric"=w766:dbl, w773:dbl, w772:dbl)
        n395 = Bundle(w737, w757, w758) -> (→"POS":cluster{dbl, dbl, dbl})  [unwired: 1 in]
        n396 = Bundle(w735, w755, w753) -> (→"RATE":cluster{dbl, dbl, dbl})  [unwired: 1 in]
        n397 = Bundle(w756, w754, w778) -> (→"ACCEL":cluster{dbl, dbl, dbl})  [unwired: 1 in]
        n398 = expression code="(x/pi)*180.0" ("radians to degrees")(w730) -> (w719:dbl)
        n399 = expression code="(x/pi)*180.0" ("radians to degrees")(w729) -> (w717:dbl)
        n400 = Initialize Array(0.0 ("element"), 26 ("dimension size")) -> (w785:dbl[])
        n401 = Multiply(x=w722, y=w720) -> (x*y=w718:dbl)
        n402 = Multiply(x=w720, y=w721) -> (x*y=w716:dbl)
        n403 = Index Array(array=w733, index #1=0 ("index")) -> (element #1=w750:dbl, element #2=w748:dbl, element #3=w749:dbl)  [unwired: 2 in]
        n404 = Select(t=w719, s=w713, f=w718) -> (s? t:f=w715:dbl)
        n405 = Select(t=w717, s=w713, f=w716) -> (s? t:f=w714:dbl)
        n406 = Replace Array Subset(array=w785, new element #1=w734, index #1=0 ("index"), new element #2=w765, new element #3=w777, new element #4=w776, new element #5=w764, new element #6=w775, new element #7=w774, new element #8=w766, new element #9=w773, new element #10=w772, new element #11=w737, new element #12=w735, new element #13=w756, new element #14=w757, new element #15=w755, new element #16=w754, new element #17=w758, new element #18=w753, new element #19=w778, new element #20=w750, new element #21=w748, new element #22=w749, new element #23=w739, new element #24=w738, new element #25=w715, new element #26=w714) -> (w784:dbl[])  [unwired: 25 in]
        n407 = shared-variable ".\\Library 1.lvlib\\output array"(w784) -> ()  [unwired: 1 in, 1 out]
        n408 = node-c288() -> ()  [unwired: 1 in, 1 out]
      }
      n409 = node-c288(w652) -> ()  [unwired: 1 out]
      n410 = Close File(refnum=w650, error in=w649) -> ()  [unwired: 2 out]
      n411 = node-c288(w666) -> ()  [unwired: 1 out]
      n412 = call "Stop_Synthesis.vi"("TCP connection ID"=w660, "error in"=w661) -> ("TCP connection ID out"=w639:refnum<k5>, "error out"=w638:errorcluster)  [unwired: 12 in]
      n413 = TCP Close Connection(connection ID=w639, error in (no error)=w638) -> (error out=w637:errorcluster)  [unwired: 1 in, 1 out]
      n414 = UDP Close(connection ID=w665, 8:w637) -> (error out=w640:errorcluster)  [unwired: 1 out]
      n415 = call <vilib>:"General Error Handler.vi"("error in (no error)"=w640) -> ()  [unwired: 2 in, 13 out]
    }
  }
  n416 = node-c288(w48) -> ()  [unwired: 1 out]
